vi "RunTest.vi"(8 "error in (no error)":errorcluster, 11 "Prueba04 in":refnum<class "Prueba04.lvclass">) -> (0 "error out":errorcluster, 2 "resultado":string, 3 "Prueba04 out":refnum<class "Prueba04.lvclass">)   [LabVIEW 2019, in "Prueba04.lvclass"]
uses:
  Prueba04.lvclass
  Control/Slide.ctl
  Prueba04.lvclass/Prueba04.ctl
  Control/SetPointGEN.ctl
  <vilib>/Utility/error.llb/DialogType.ctl
  QMH/Message Queue/Enqueue Message (Single).vi
  <vilib>/Utility/error.llb/Error Cluster From Error Code.vi
  <vilib>/ErrorRing/Error Ring.xnode
  Prueba/Prueba.lvclass
  QMH/User Event - Stop/User Event - Stop.lvlib
  QMH/Message Queue/Message Queue.lvlib
panel:
  out "frecZ1":dbl
  out "frecC1":dbl
  out "fila actual Z":i32
  out "frec_generar_Z2":string
  out "volt_generar_Z2":string
  out "frec_ref_Z_2":string="inicio"
  out "Vref_Z":dbl
  out "IndicadorAjuste_Z":dbl caption="Ajuste de amplitud [mV]"
  out "cumple_no_cumple_Z":bool
  out "cumple_no_cumple_C":bool
  out "fila actual C":i32
  out "frec_generar_C2":string
  out "volt_generar_C2":string
  out "frec_ref_C":string="inicio"
  out "IndicadorAjuste_C":dbl caption="Ajuste de amplitud [mV]"
  out "Vref_C":dbl
  out "cumple_no_cumple_A":bool
  out "ponderacion_Z":bool
  out "ponderacion_C":bool
  out "volt_generar_A2":string
  out "Vref_A 2":dbl
  out "frecA1":dbl
  out "frec_generar_C2":string
  out "Voltajes_Ref_Z":string[](array[string])
  out "Voltajes_Ref_C":string[](array[string])
  out "fila actual Z":i32
  out "fila actual C":i32
  out "frec_ref_Z":string="inicio"
  out "frec_ref_C":string="inicio"
  out "frec_generar_A2":string
  out "fila actual A":i32
  out "Voltajes_Ref_A":string[](array[string])
  out "frec_ref_A":string="inicio"
  out "Vref_A":dbl
  out "IndicadorAjuste_A":dbl caption="Ajuste de amplitud [mV]"
  out "ponderacion_A":bool
  out "Tab":T1(tab)
  in  "go_A":bool
  in  "go_C":bool
  in  "go_Z":bool
  in  "seguir":bool
  out "no_cumple_prueba04":bool
  out "cumple_prueba04":bool
  out "estado_ensayo_A":string="Ensayo ya realizado"
  out "estado_ensayo_C":string="Ensayo ya realizado"
  out "estado_ensayo_Z":string="Ensayo ya realizado"
  in  "cb_frec_A_1":string(combo)="1000"
  in  "guardar_Vref_A":bool
  out "niveldBA_1":dbl=95.0
  out "rangoRefA_1":dbl=140.0
  in  "generarA1":bool
  in  "VoltAjuste_A":T2=20.0 caption="Ajuste de amplitud [mV]" scale=0.0..50.0
  out "voltMonA_1":dbl format="%.5f"
  out "frecMonA_1":dbl format="%#.1f"
  in  "ir a resultados_A":bool
  out "Pict Ring_2":u16(ring)
  out "Pict Ring_1":u16(ring)
  in  "cb_frec_A_2":string(combo)="31,5"
  out "voltaje_A":dbl
  in  "generarA2":bool
  out "cumple_A":bool
  out "no_cumple_A":bool
  in  "ir a inicio desde A":bool
  in  "Tabla_A":string[][](table)
  out "voltMonA_2":dbl format="%.5f"
  out "frecMonA_2":dbl format="%#.1f"
  in  "cb_frec_C_1":string(combo)="1000"
  in  "guardar_Vref_C":bool
  out "niveldBC_1":dbl
  out "rangoRefC_1":dbl
  in  "generarC1":bool
  in  "VoltAjuste_C":T2=20.0 caption="Ajuste de amplitud [mV]" scale=0.0..50.0
  out "voltMonC_1":dbl
  out "frecMonC_1":dbl
  in  "ir a resultados_C":bool
  in  "cb_frec_C_2":string(combo)="31,5"
  out "voltaje_C":dbl
  in  "generarC2":bool
  out "voltMonC_2":dbl
  out "frecMonC_2":dbl
  in  "Tabla_C":string[][](table)
  in  "ir a inicio desde C":bool
  out "cumple_C":bool
  out "no_cumple_C":bool
  out "Pict Ring_1 2":u16(ring)
  out "Pict Ring_2 2":u16(ring)
  in  "cb_frec_Z_1":string(combo)="1000"
  out "niveldBZ_1":dbl
  out "rangoRefZ_1":dbl
  in  "generarZ1":bool
  in  "VoltAjuste_Z":T2=20.0 caption="Ajuste de amplitud [mV]" scale=0.0..200.0
  out "voltMonZ_1":dbl
  out "frecMonZ_1":dbl
  in  "ir a resultados _Z":bool
  in  "guardar_Vref_Z":bool
  out "Pict Ring_2 3":u16(ring)
  out "Pict Ring_1 3":u16(ring)
  in  "cb_frec_Z_2":string(combo)="31,5"
  out "voltaje_Z":dbl
  in  "generarZ2":bool
  in  "ir a inicio desde Z":bool
  in  "Tabla_Z":string[][](table)
  out "voltMonZ_2":dbl
  out "frecMonZ_2":dbl
  out "cumple_Z":bool
  out "no_cumple_Z":bool
  # "Cumple"
  # "No Cumple"
  # "Ensayo Eléctrico Ponderación A"
  # "Ensayo Eléctrico Ponderación C"
  # "Ensayo Eléctrico Ponderación Z"
  # "Ensayo Eléctrico Ponderación A – Selección de Señal de referencia"
  # "Elección Señal de Referencia\nsegún marca y modelo de sonómetro"
  # "Nivel en dB"
  # "Rango Referencia"
  # "Frecuencia"
  # "Monitoreo"
  # "Frecuencia"
  # "Hz"
  # "Voltaje"
  # "V"
  # "Ensayo Eléctrico Ponderación A – Tabla de Resultados"
  # "Cumple"
  # "No Cumple"
  # "Hz"
  # "mV"
  # "Voltaje"
  # "Frecuencia"
  # "Ponderación A"
  # "Monitoreo"
  # "Frecuencia"
  # "Hz"
  # "Voltaje"
  # "V"
  # "Ensayo Eléctrico Ponderación C – Selección de Señal de referencia"
  # "Elección Señal de Referencia\nsegún marca y modelo de sonómetro"
  # "Nivel en dB"
  # "Rango Referencia"
  # "Frecuencia"
  # "Monitoreo"
  # "Frecuencia"
  # "Hz"
  # "Voltaje"
  # "V"
  # "Ensayo Eléctrico Ponderación C – Tabla de Resultados"
  # "Cumple"
  # "No Cumple"
  # "Hz"
  # "mV"
  # "Voltaje"
  # "Frecuencia"
  # "Monitoreo"
  # "Frecuencia"
  # "Hz"
  # "Voltaje"
  # "V"
  # "Ponderación C"
  # "Ensayo Eléctrico Ponderación Z – Selección de Señal de referencia"
  # "Elección Señal de Referencia\nsegún marca y modelo de sonómetro"
  # "Nivel en dB"
  # "Rango Referencia"
  # "Frecuencia"
  # "Monitoreo"
  # "Frecuencia"
  # "Hz"
  # "Voltaje"
  # "V"
  # "Ensayo Eléctrico Ponderación Z – Tabla de Resultados"
  # "Cumple"
  # "No Cumple"
  # "Hz"
  # "mV"
  # "Voltaje"
  # "Frecuencia"
  # "Ponderación Z"
  # "Monitoreo"
  # "Frecuencia"
  # "Hz"
  # "Voltaje"
  # "V"
  # "4. Ensayo  de las ponderaciones frecuenciales con señales eléctricas. IEC 61672-3: 2006 Cláusula 12"
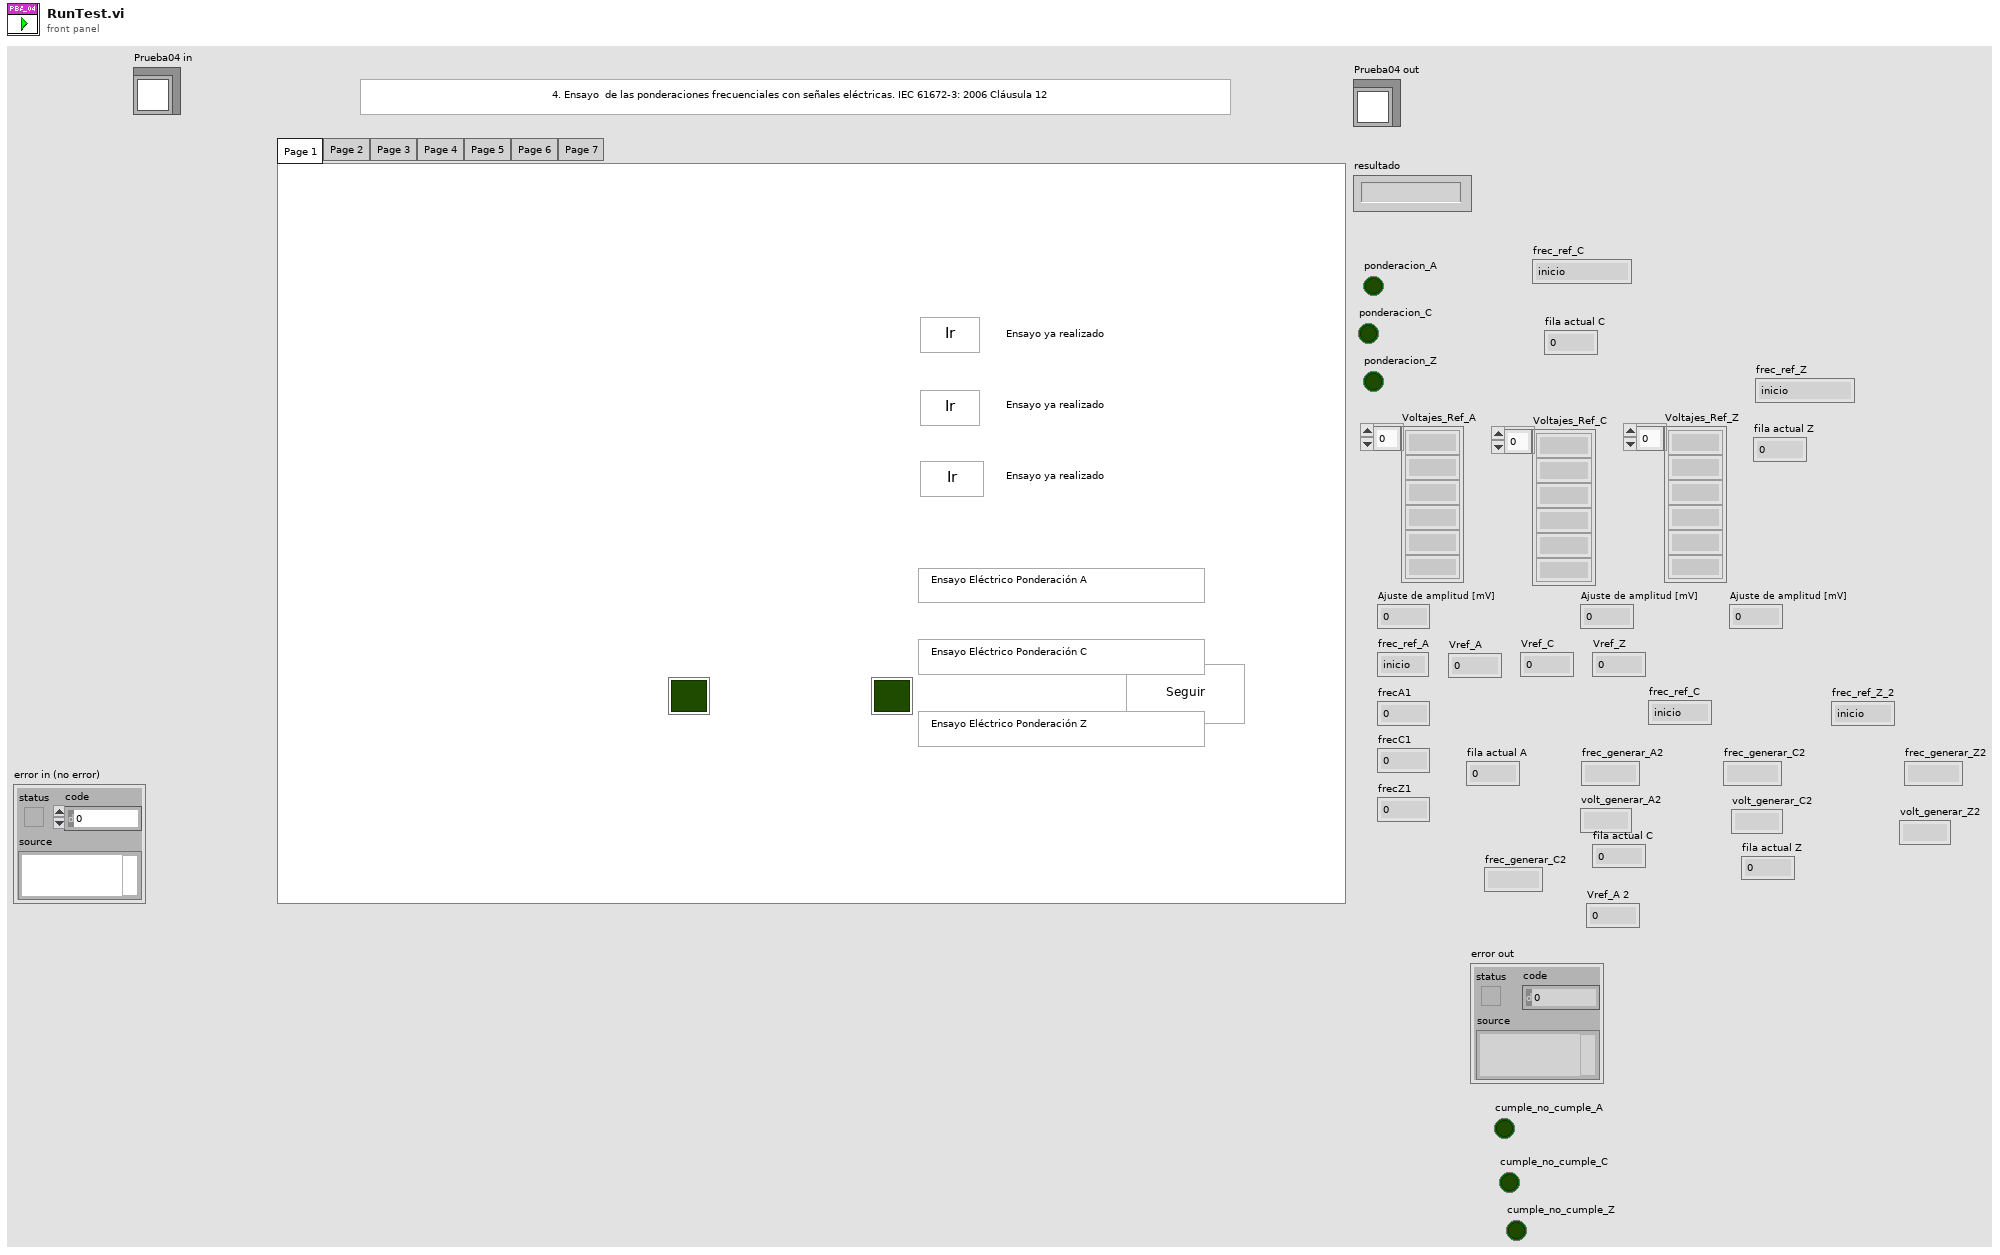
[diagram p1: front panel]
types:
  T1 = enum32{"Page 1", "Page 2", "Page 3", "Page 4", "Page 5", "Page 6", "Page 7"}
  T2 = typedef "Prueba04.lvclass/Slide.ctl" = dbl
  T3 = enum8{"Enabled", "Disabled", "Disabled and Grayed Out"}
  T4 = typedef "Message Queue.lvlib/All Message Queues.ctl" = cluster{"MHL":refnum<queue>, "Inst_CNT90":refnum<queue>, "Inst_DS360":refnum<queue>, "Inst_Keithley2002":refnum<queue>, "Inst_DAQ":refnum<queue>, "BD":refnum<queue>, "Pistofono":refnum<queue>, "Nexus":refnum<queue>}
  T5 = typedef "Prueba04.lvclass/SetPointGEN.ctl" = cluster{"frec":dbl, "amp":dbl, "letra":string}
  T6 = cluster{"ControlName":string, "ControlReference":refnum<vi>}[]
  T7 = cluster{"Medido":dbl, "Error":dbl, "Ref":dbl, "Incert_exp":dbl, "Tol+":dbl, "Tol-":dbl, "fila":i32}
  T8 = typedef "DialogType.ctl" = u16
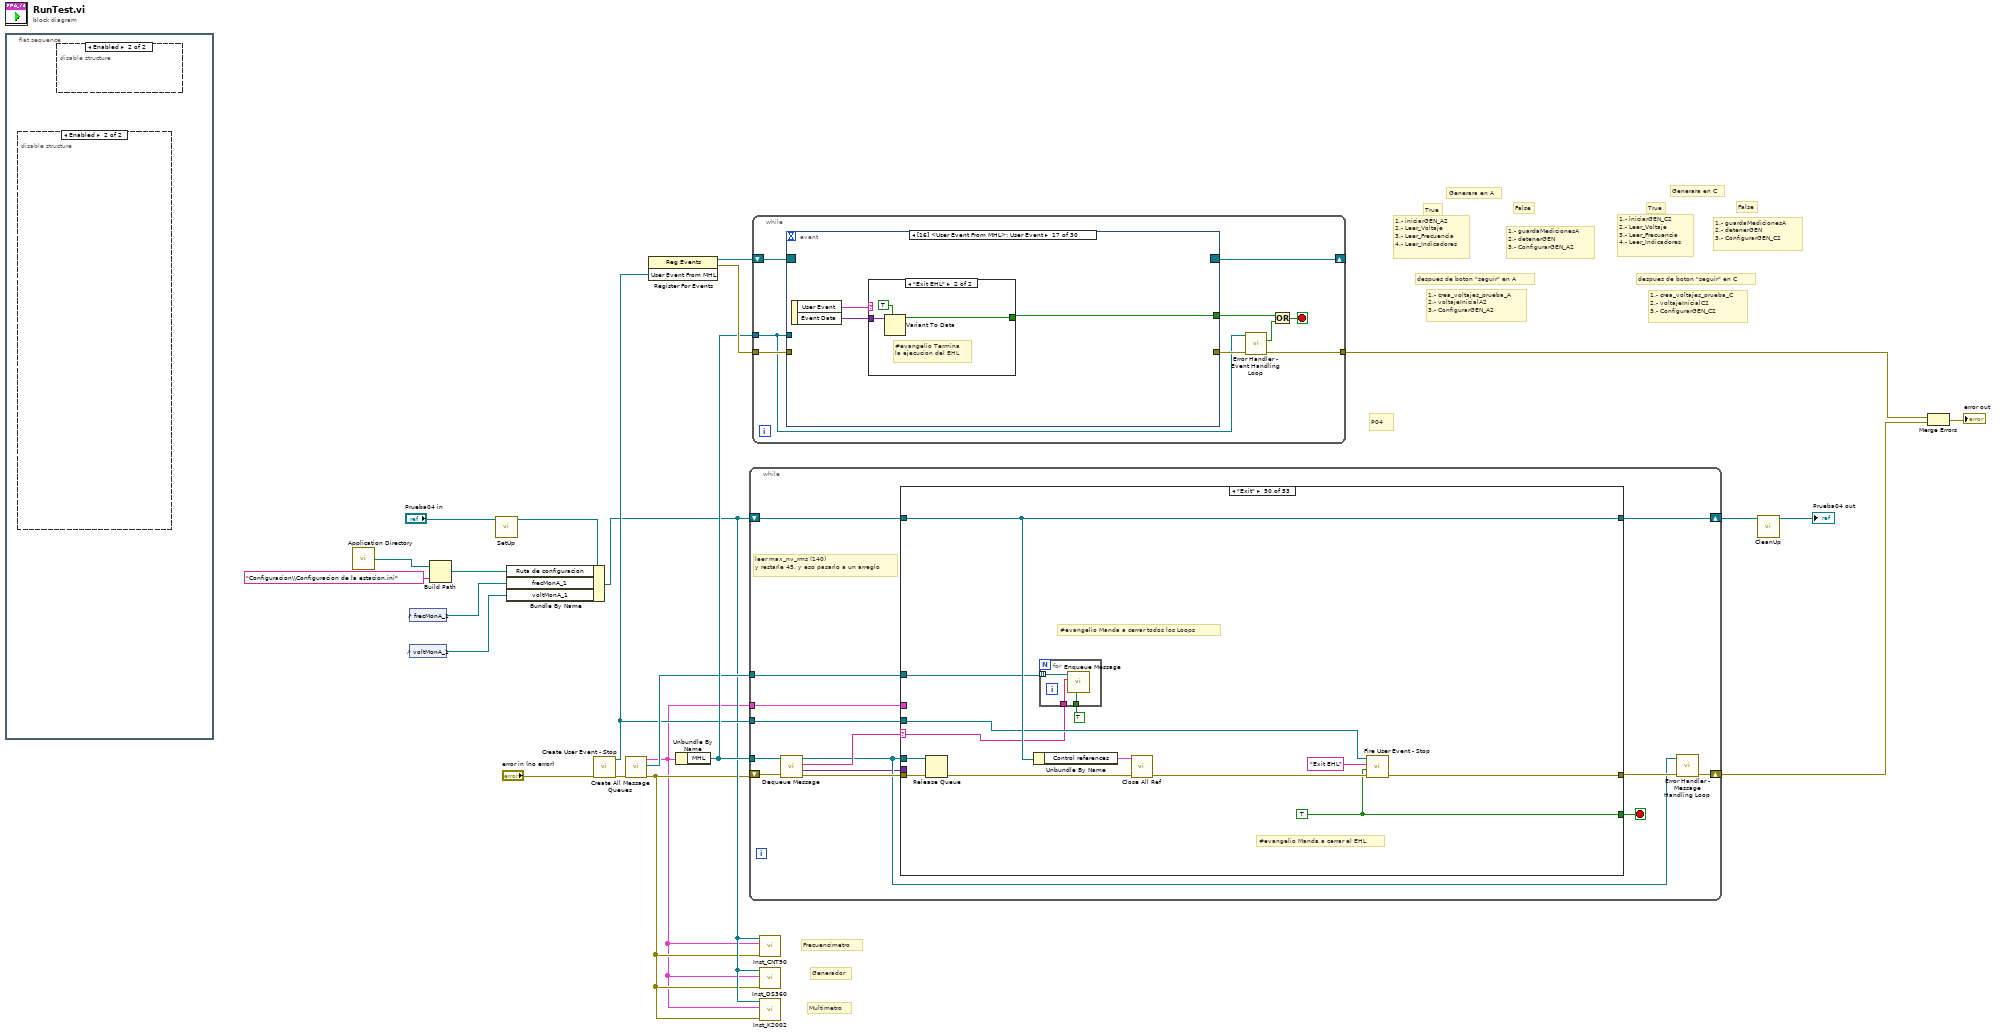
[diagram p0: block diagram]
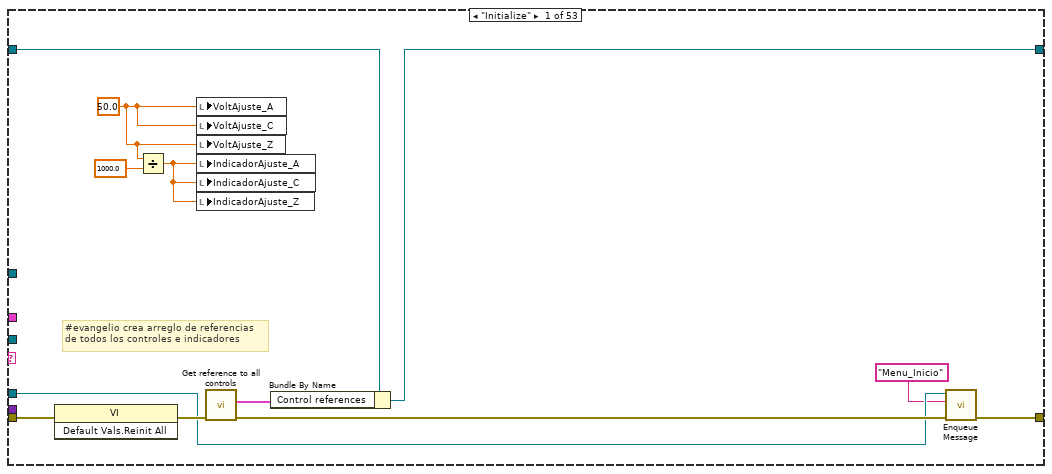
[diagram p2: hidden frame]
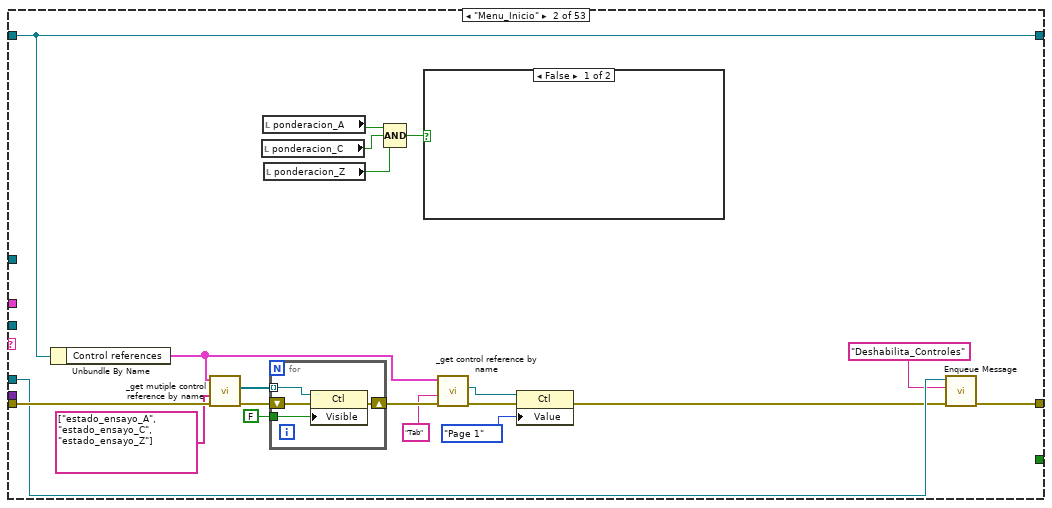
[diagram p3: hidden frame]
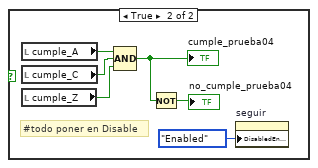
[diagram p4: hidden frame]
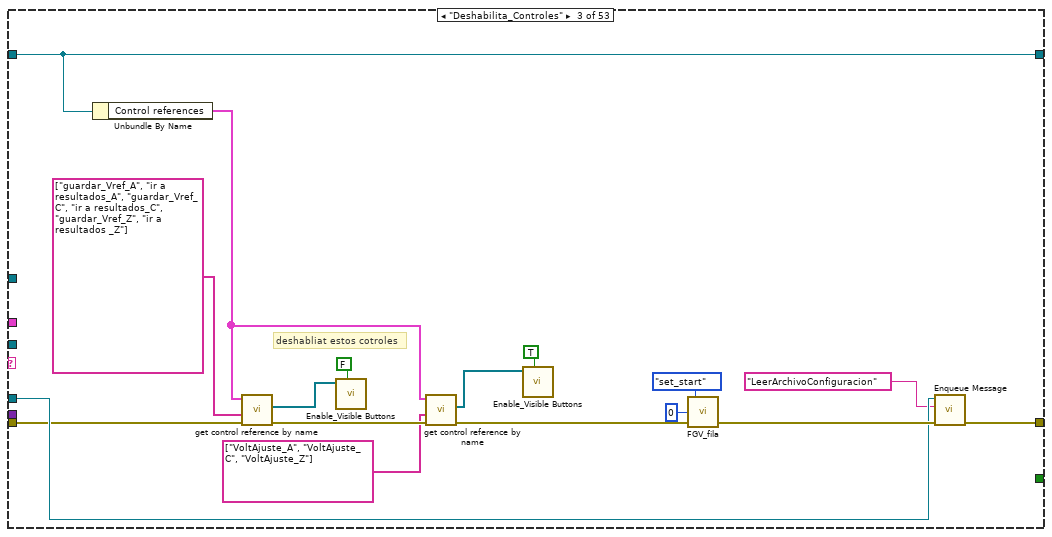
[diagram p5: hidden frame]
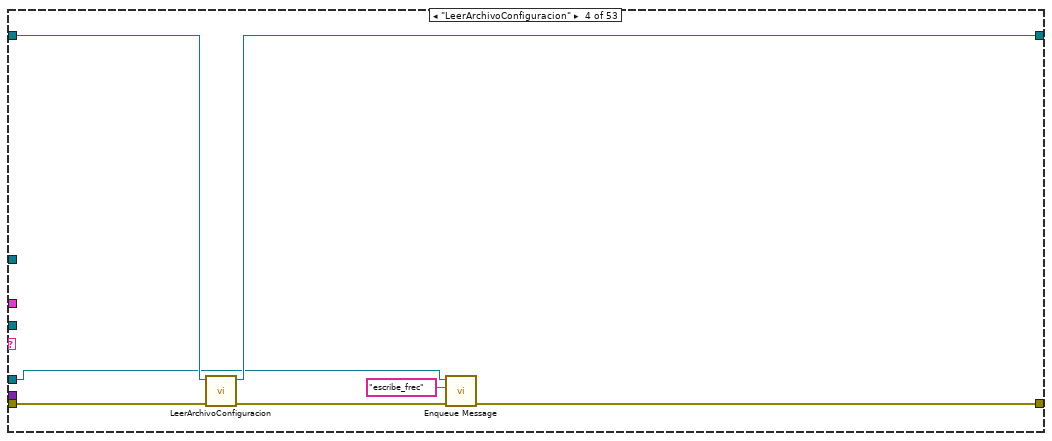
[diagram p6: hidden frame]
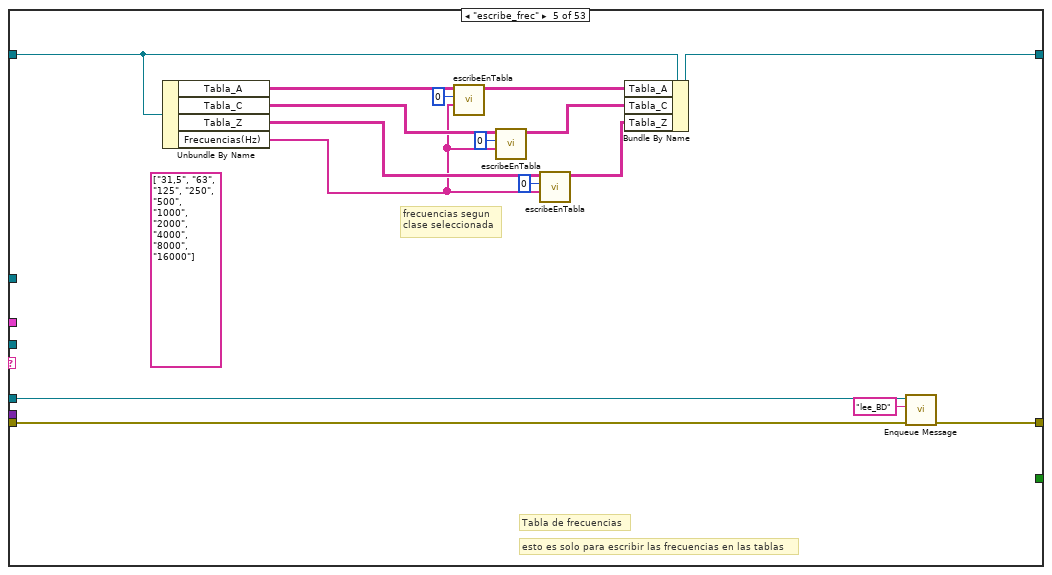
[diagram p7: hidden frame]
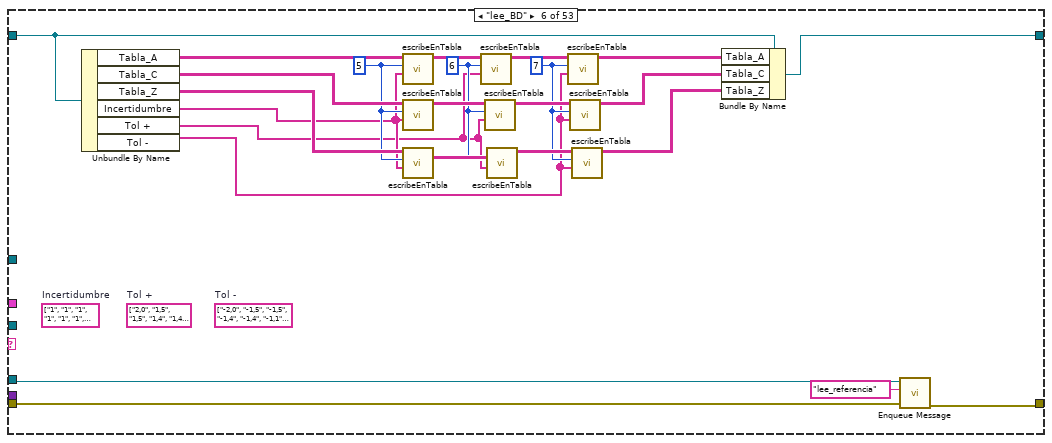
[diagram p8: hidden frame]
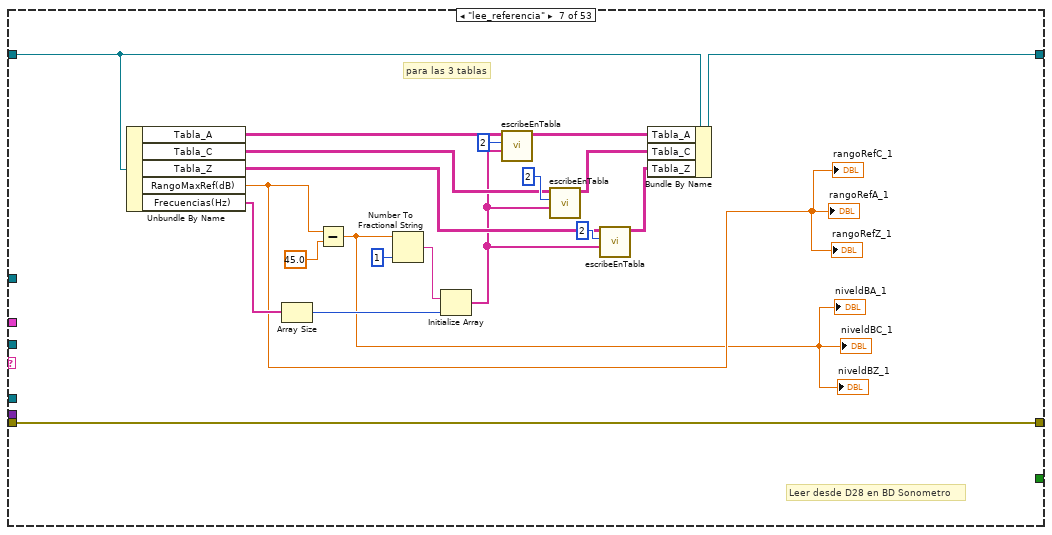
[diagram p9: hidden frame]
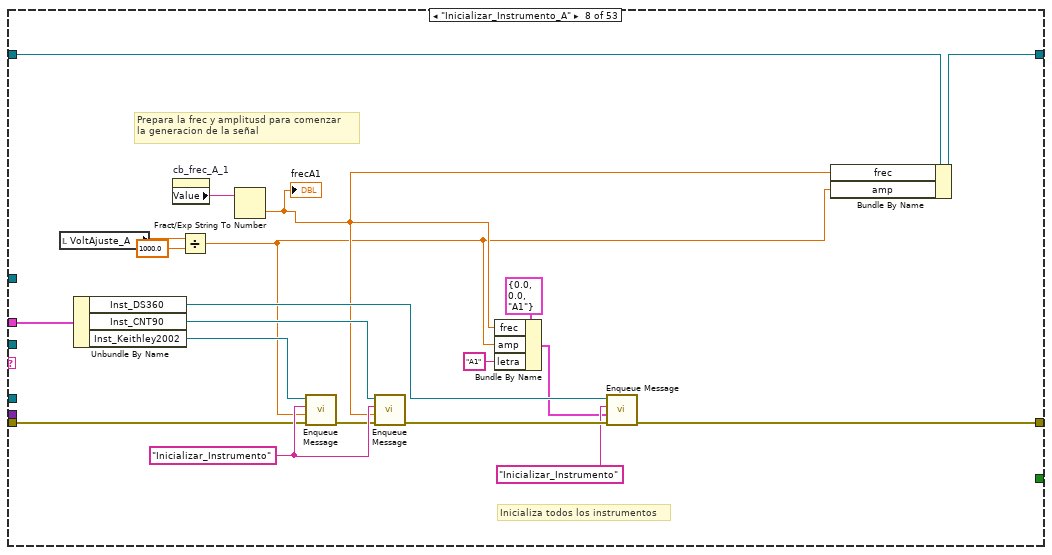
[diagram p10: hidden frame]
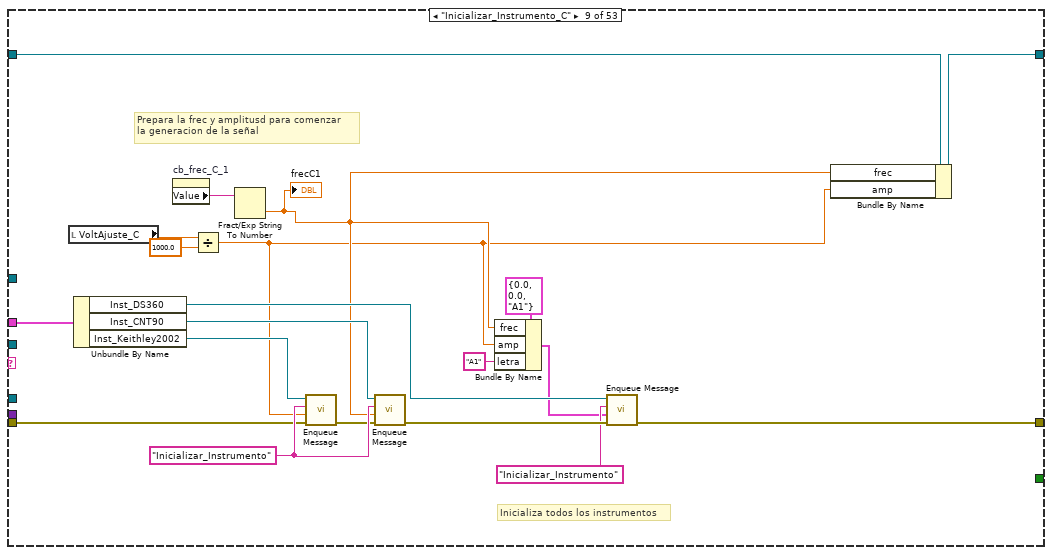
[diagram p11: hidden frame]
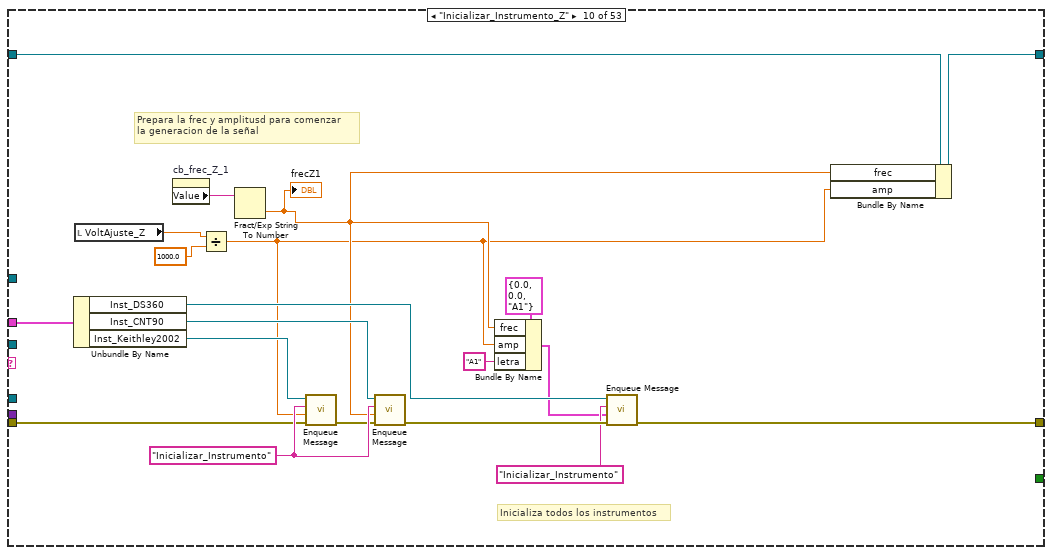
[diagram p12: hidden frame]
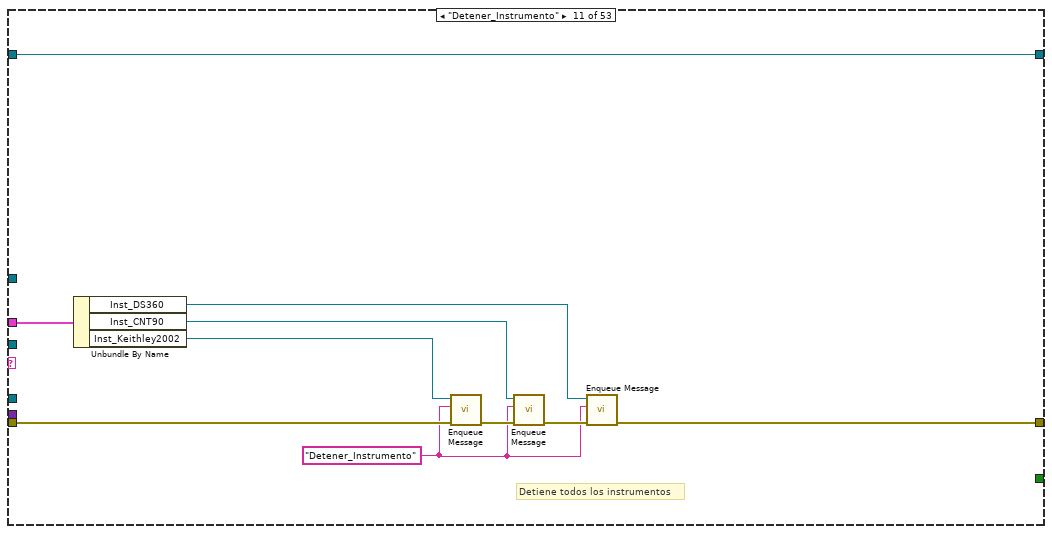
[diagram p13: hidden frame]
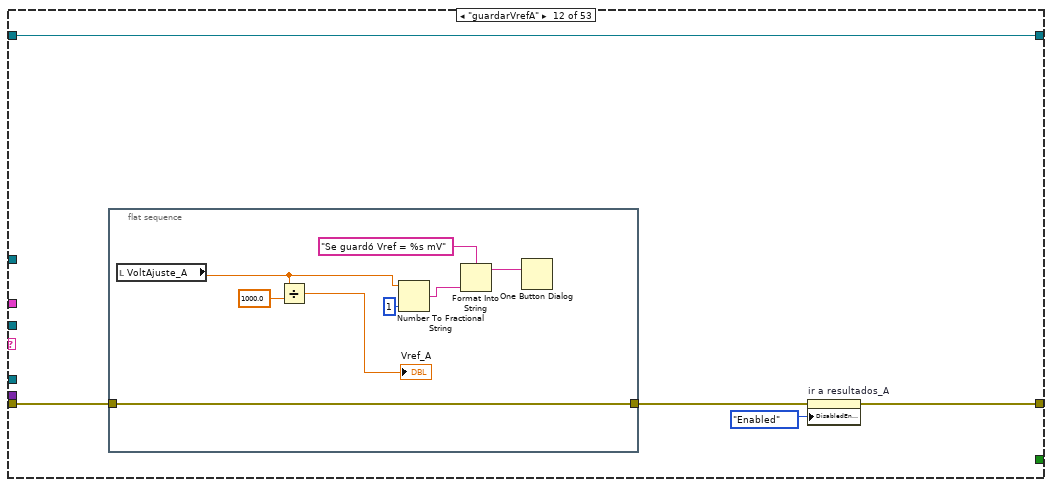
[diagram p14: hidden frame]
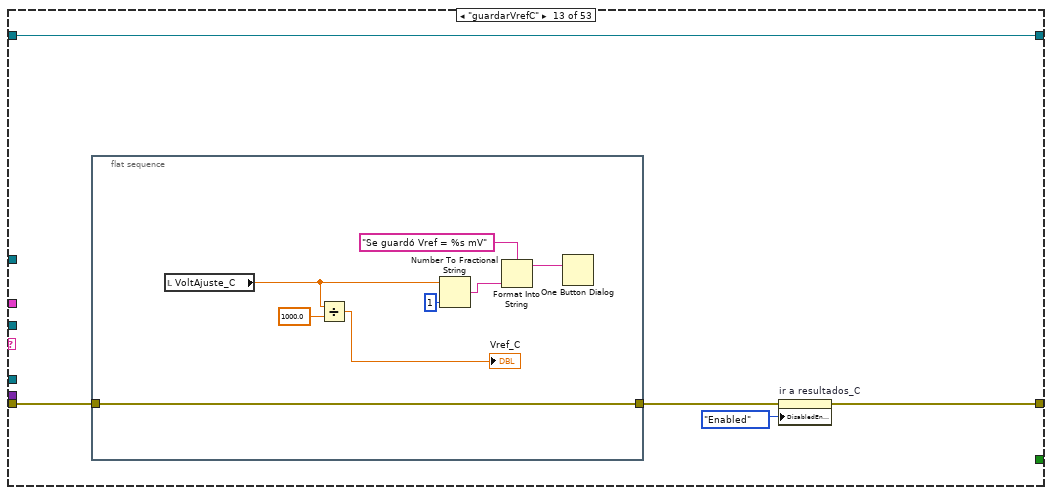
[diagram p15: hidden frame]
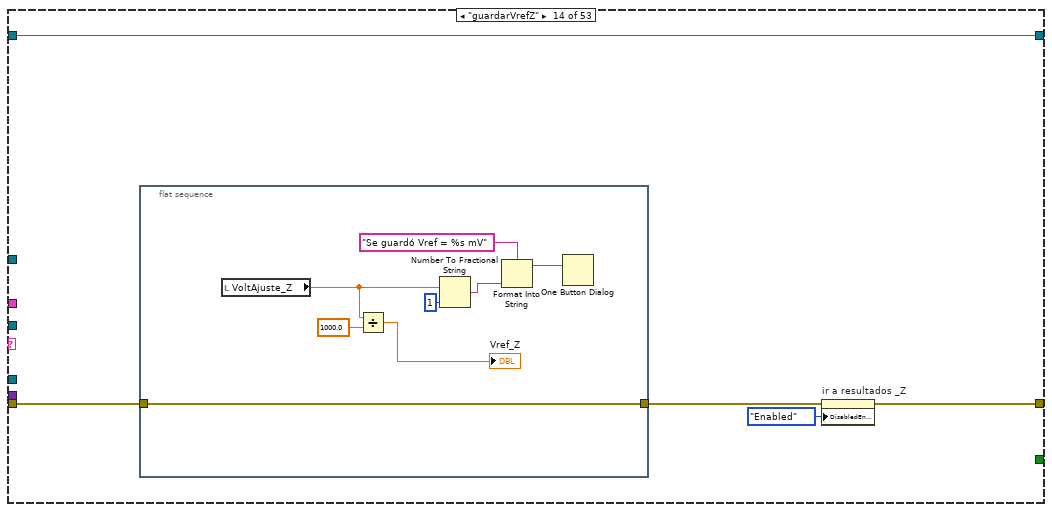
[diagram p16: hidden frame]
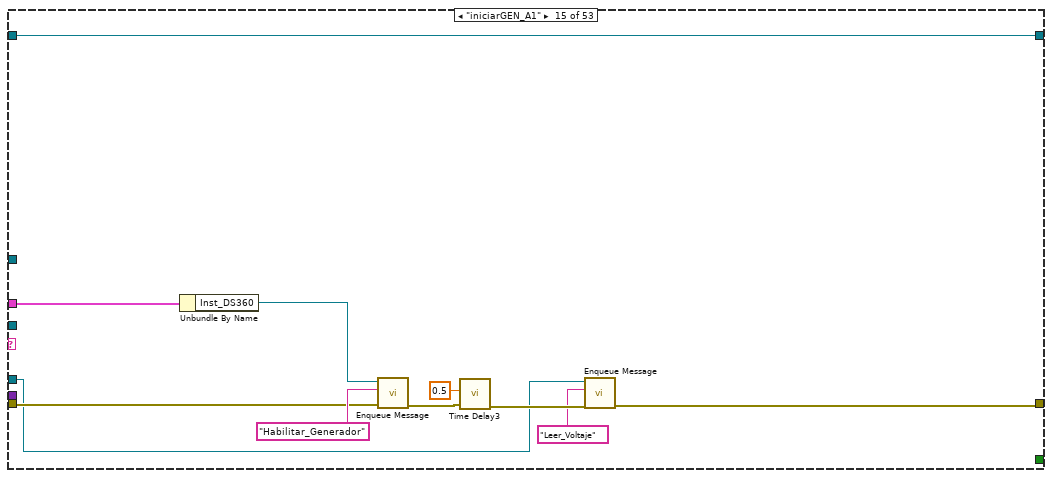
[diagram p17: hidden frame]
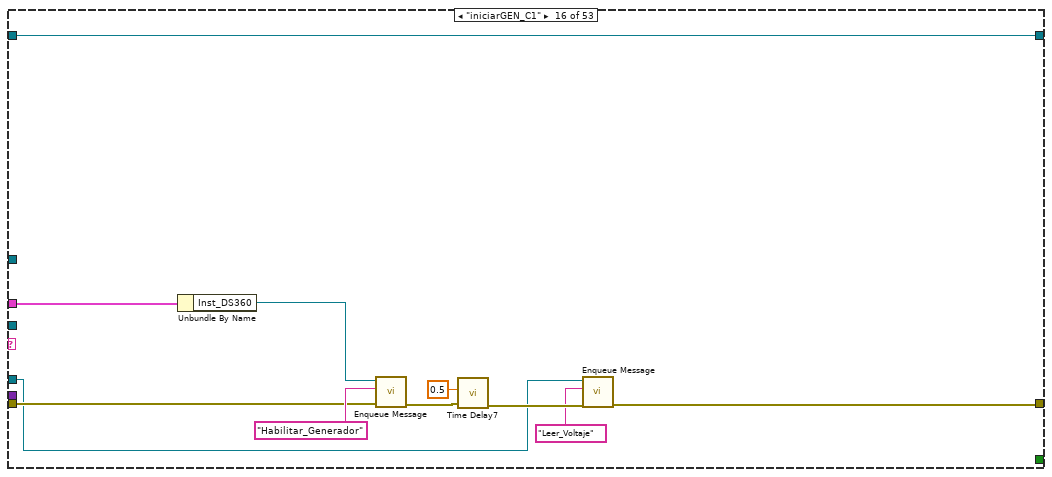
[diagram p18: hidden frame]
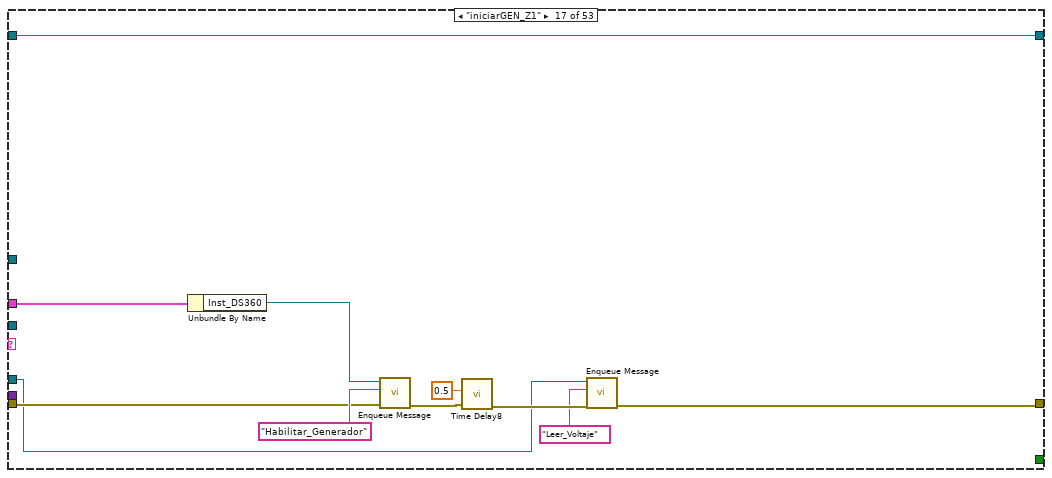
[diagram p19: hidden frame]
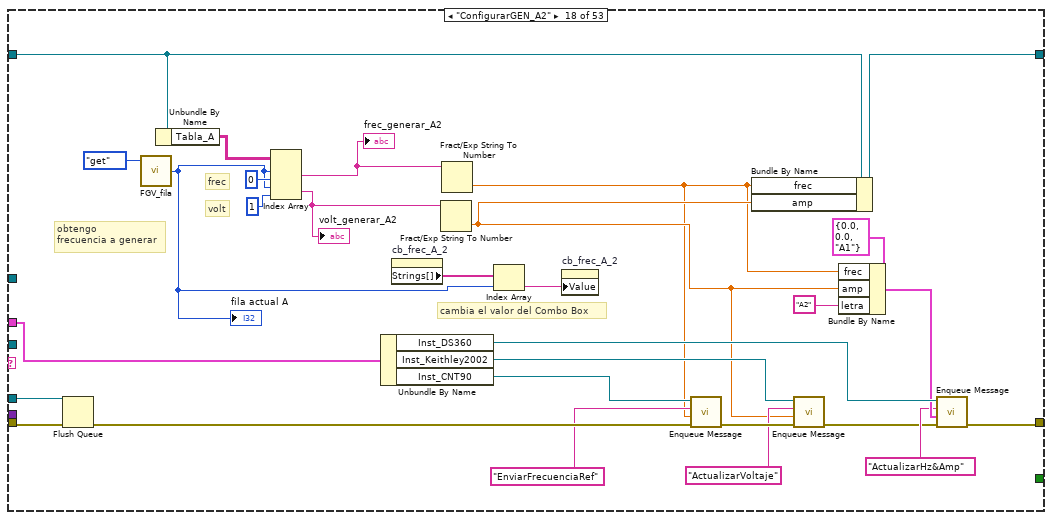
[diagram p20: hidden frame]
diagram:
  # "despues de boton \"seguir\" en C"
  # "1.- crea_voltajes_prueba_C\n2.- voltajeInicialC2\n3.- ConfigurarGEN_C2"
  # "1.- guardaMedicionesA\n2.- detenerGEN\n3.- ConfigurarGEN_A2"
  # "False"
  # "True"
  # "1.- iniciarGEN_A2\n2.- Leer_Voltaje\n3.- Leer_Frecuencia\n4.- Leer_Indicadores"
  # "Generara en A"
  # "1.- guardaMedicionesA\n2.- detenerGEN\n3.- ConfigurarGEN_C2"
  # "False"
  # "True"
  # "1.- iniciarGEN_C2\n2.- Leer_Voltaje\n3.- Leer_Frecuencia\n4.- Leer_Indicadores"
  # "Generara en C"
  # "despues de boton \"seguir\" en A"
  # "1.- crea_voltajes_prueba_A\n2.- voltajeInicialA2\n3.- ConfigurarGEN_A2"
  # "P04"
  # "Multimetro"
  # "Generador"
  # "Frecuencimetro"
  n1 = flat-sequence {
    frame #0 {
      n2 = disable-structure shown="Enabled" {
        frame Disabled {
          w24 = FALSE ("cumple_A")
          n3 = local write "generarA1"(w24) -> ()
          n4 = local write "no_cumple_A"(w24) -> ()
          n5 = local write "cumple_prueba04"(w24) -> ()
          n6 = local write "no_cumple_prueba04"(w24) -> ()
          n7 = local write "generarA2"(w24) -> ()
          n8 = local write "generarZ1"(w24) -> ()
          n9 = local write "no_cumple_Z"(w24) -> ()
          n10 = local write "generarC1"(w24) -> ()
          n11 = local write "no_cumple_C"(w24) -> ()
          n12 = local write "generarC2"(w24) -> ()
          n13 = local write "generarZ2"(w24) -> ()
          n14 = local write "ponderacion_A"(w24) -> ()
          n15 = local write "ponderacion_C"(w24) -> ()
          n16 = local write "ir a inicio desde C"(w24) -> ()
          n17 = local write "ponderacion_Z"(w24) -> ()
          n18 = local write "cumple_A"(w24) -> ()
          n19 = local write "cumple_C"(w24) -> ()
          n20 = local write "cumple_Z"(w24) -> ()
          n21 = local write "ir a inicio desde A"(w24) -> ()
          n22 = local write "ir a inicio desde Z"(w24) -> ()
        }
        frame Enabled {
        }
      }
      n23 = disable-structure shown="Enabled" {
        frame Disabled {
          n24 = property on="seguir" class="Bool"("DisabledEnum"=T3."Enabled" ("Disabled")) -> ()  [unwired: 2 in, 2 out]
        }
        frame Enabled {
        }
      }
    }
  }
  n25 = call <vilib>:"Application Directory.vi"() -> ("Application Directory"=w16:path)
  n26 = control-ref of="frecMonA_1"() -> (w2:refnum<vi>)
  n27 = control-ref of="voltMonA_1"() -> (w1:refnum<vi>)
  n28 = Build Path(base path=w16, name or relative path="Configuracion\\Configuracion de la estacion.ini") -> (appended path=w15:path)
  n29 = call-dynamic "SetUp.vi"("Prueba04 in"="Prueba04 in") -> ("Prueba04 out"=w14:refnum<class "Prueba04.lvclass">)  [unwired: 9 in, 1 out]
  n30 = Bundle By Name(cluster=w14, "Ruta de configuracion"=w15, "frecMonA_1"=w2, "voltMonA_1"=w1) -> (w5:refnum<class "Prueba04.lvclass">)
  n31 = call "Create User Event - Stop.vi"("error in (no error)"="error in (no error)") -> ("error out"=w13:errorcluster, "User Event From MHL"=w6:refnum<user-event>)  [unwired: 9 in]
  n32 = call "Create All Message Queues.vi"("error in (no error)"=w13) -> ("error out"=w4:errorcluster, "PL Queues Array"=w7:refnum<queue>[], "All Message Queues out"=w3:T4)  [unwired: 8 in]
  n33 = register-events(w6) -> (reference out=w18:refnum<event-registration>, error out=w11:errorcluster)  [unwired: 2 in]
  n34 = Unbundle By Name(w3) -> ("MHL"=w10:refnum<queue>)
  n35 = while {
    shift-right: [w35] -> w19
    shift-left: w5 -> [w36]
    shift-right: [w30] -> w21
    shift-left: w4 -> [w34]
    tunnel: w10 -> [w33]
    tunnel: w7 -> [w27]
    tunnel: w3 -> [w26]
    tunnel: w6 -> [w25]
    stop <- w37 stop-if-true
    # "leer max_nv_rms (140)\ny restarle 45, y eso pasarlo a un arreglo"
    n36 = call "Dequeue Message.vi"("error in (no error)"=w34, "Message Queue"=w33) -> ("error out"=w38:errorcluster, "Message Data"=w28:variant, "Message"=w32:string, "dup Message Queue"=w29:refnum<queue>)  [unwired: 6 in]
    n37 = case shown="\"Exit\"" w32 {
      selector: w32 -> [_ _ _ _ _ _ _ _ _ _ _ _ _ _ _ _ _ _ _ _ _ _ _ _ _ _ _ _ _ _ _ _ _ _ _ _ _ _ _ _ _ _ _ _ _ _ _ _ _ w1001 _ w1026 _]
      tunnel: [_ _ _ _ _ _ _ _ _ _ _ _ _ _ _ _ _ _ _ _ _ _ _ _ _ _ _ _ _ _ _ _ _ _ _ _ _ _ _ _ _ _ _ _ _ _ _ _ _ w1000 _ _ _] -> w37
      tunnel: [w47 w69 w95 w100 w120 w144 w164 w173 w193 w213 w232 w235 w248 w261 w275 w286 w297 w322 w348 w375 w393 w405 w417 w428 w441 w459 w468 w494 w500 w522 w545 w568 w578 w590 w602 w611 w620 w627 w646 w665 w684 w727 w814 w850 w863 w903 w943 w981 w983 w999 w1016 w1025 w1036] -> w31
      tunnel: w38 -> [w49 w70 w91 w104 w119 w143 w164 w170 w190 w210 w234 w238 w251 w264 w277 w288 w299 w329 w356 w385 w396 w408 w420 w431 w444 w461 w470 w486 w507 w531 w554 w570 w581 w591 w603 w612 w621 w637 w656 w675 w695 w728 w815 w850 w864 w904 w944 w978 w984 w1006 w1018 _ w1036]
      tunnel: w36 -> [w46 w56 w90 w103 w108 w142 w161 w183 w203 w223 w233 w239 w252 w265 w284 w295 w306 w327 w353 w383 w403 w415 w427 w440 w453 w458 w483 w493 w503 w525 w548 w569 w579 w589 w597 w606 w615 w635 w654 w673 w689 w723 w810 w843 w859 w899 w939 w976 w990 w1004 w1024 w1027 w1035]
      tunnel: [w45 w56 w90 w102 w112 w138 w162 w182 w202 w222 w233 w239 w252 w265 w284 w295 w306 w328 w354 w384 w403 w415 w427 w440 w453 w458 w483 w493 w505 w527 w550 w569 w579 w589 w597 w606 w615 w633 w652 w671 w690 w723 w810 w843 w857 w897 w937 w976 w990 w1004 w1024 w1027 w1035] -> w35
      tunnel: w29 -> [w44 w68 w93 w99 w106 w122 _ _ _ _ _ _ _ _ w274 w285 w296 w323 w349 w379 w394 w406 w418 w430 w443 w460 _ _ w501 w523 w546 w567 w577 w587 _ _ _ w629 w648 w667 w683 w721 w808 _ w853 w893 w933 w975 w985 w1005 w1017 _ _]
      tunnel: w28 -> [_ _ _ _ _ _ _ _ _ _ _ _ _ _ _ _ _ _ _ _ _ _ _ _ _ _ w467 _ _ _ _ _ _ _ _ _ _ w628 w647 w666 w685 w722 w809 _ _ _ _ _ _ _ w1015 _ _]
      tunnel: w27 -> [_ _ _ _ _ _ _ _ _ _ _ _ _ _ _ _ _ _ _ _ _ _ _ _ _ _ _ _ _ _ _ _ _ _ _ _ _ _ _ _ _ _ _ _ _ _ _ _ _ w1003 _ _ _]
      tunnel: w26 -> [_ _ _ _ _ _ _ w181 w201 w221 w231 _ _ _ w276 w287 w298 w321 w347 w374 w395 w407 w419 w429 w442 _ w469 w485 _ _ _ _ _ _ _ _ _ _ _ _ _ _ _ _ _ _ _ _ _ _ _ _ _]
      tunnel: w25 -> [_ _ _ _ _ _ _ _ _ _ _ _ _ _ _ _ _ _ _ _ _ _ _ _ _ _ _ _ _ _ _ _ _ _ _ _ _ _ _ _ _ _ _ _ _ _ _ _ _ w1002 _ _ _]
      frame "Initialize" {
        w39 = T2 50.0 ("VoltAjuste_A")
        # "#evangelio crea arreglo de referencias\nde todos los controles e indicadores"
        n38 = invoke class="VI" method="Default Vals.Reinit All"(error in=w49) -> (error out=w50:errorcluster)  [unwired: 2 in, 2 out]
        n39 = Divide(x=w39, y=T2 1000.0) -> (x/y=w41:T2)
        n40 = local write "VoltAjuste_A"(w39) -> ()
        n41 = local write "VoltAjuste_C"(w39) -> ()
        n42 = local write "VoltAjuste_Z"(w39) -> ()
        n43 = local write "IndicadorAjuste_A"(w41) -> ()
        n44 = local write "IndicadorAjuste_C"(w41) -> ()
        n45 = local write "IndicadorAjuste_Z"(w41) -> ()
        n46 = call "Get reference to all controls.vi"("error in (no error)"=w50) -> ("error out"=w48:errorcluster, "Control references"=w42:T6)  [unwired: 5 in]
        n47 = Bundle By Name(cluster=w46, "Control references"=w42) -> (w45:refnum<class "Prueba04.lvclass">)
        n48 = call-poly "Enqueue Message.vi"("error in (no error)"=w48, "Message"="Menu_Inicio", "Message Queue"=w44) -> ("error out"=w47:errorcluster)  [unwired: 7 in, 1 out]
      }
      frame "Menu_Inicio" {
        n49 = Unbundle By Name(w56) -> ("Control references"=w55:T6)
        n50 = call "_get mutiple control reference by name.vi"("error in (no error)"=w70, "Control names"=string[] ["estado_ensayo_A", "estado_ensayo_C", "estado_ensayo_Z"], "Control references"=w55) -> ("error out"=w66:errorcluster, "References"=w64:refnum<vi>[])  [unwired: 3 in]
        n51 = local read "ponderacion_C"() -> (w52:bool)
        n52 = local read "ponderacion_A"() -> (w53:bool)
        n53 = local read "ponderacion_Z"() -> (w54:bool)
        n54 = for {
          shift-right: [w79] -> w62
          shift-left: w66 -> [w80]
          tunnel: w64 -> [w78] mode=indexing
          tunnel: FALSE -> [w77]
          n55 = property class="Ctl"(reference=w78, error in=w80, "Visible"=w77) -> (error out=w79:errorcluster)  [unwired: 1 out]
        }
        n56 = Compound Arithmetic op=AND(w53, w52, w54) -> (w51:bool)
        n57 = case shown="False" w51 {
          frame False {
          }
          frame True {
            # "#todo poner en Disable"
            n58 = local read "cumple_A"() -> (w76:bool)
            n59 = local read "cumple_C"() -> (w72:bool)
            n60 = local read "cumple_Z"() -> (w71:bool)
            n61 = Compound Arithmetic op=AND(w76, w72, w71) -> (w73:bool)
            "cumple_prueba04" <- w73
            n62 = Not(x=w73) -> (.not. x?=→"no_cumple_prueba04":bool)
            n63 = property on="seguir" class="Bool"("DisabledEnum"=T3."Enabled" ("Disabled")) -> ()  [unwired: 2 in, 2 out]
          }
        }
        n64 = call "_get control reference by name.vi"("error in (no error)"=w62, "Control name"="Tab" ("Message"), "Control references"=w55) -> ("error out"=w61:errorcluster, "Ctl Refnum"=w58:refnum<vi>)  [unwired: 3 in]
        n65 = property class="Ctl"(reference=w58, error in=w61, "Value"=T1."Page 1" ("Tab_Prueba04")) -> (error out=w59:errorcluster)  [unwired: 1 out]
        n66 = call-poly "Enqueue Message.vi"("error in (no error)"=w59, "Message"="Deshabilita_Controles", "Message Queue"=w68) -> ("error out"=w69:errorcluster)  [unwired: 7 in, 1 out]
      }
      frame "Deshabilita_Controles" {
        # "deshabliat estos cotroles"
        n67 = Unbundle By Name(w90) -> ("Control references"=w86:T6)
        n68 = call-poly "get control reference by name.vi"("error in (no error)"=w91, "Control names"=string[] ["guardar_Vref_A", "ir a resultados_A", "guardar_Vref_C", "ir a resultados_C", "guardar_Vref_Z", "ir a resultados _Z"] ("Message"), "Control references"=w86) -> ("error out"=w85:errorcluster, "References"=w88:refnum<vi>[])  [unwired: 3 in]
        n69 = call "Enable_Visible Buttons.vi"("Enable? (T)"=FALSE, "Controls Ref Array"=w88) -> ()  [unwired: 10 in]
        n70 = call-poly "get control reference by name.vi"("error in (no error)"=w85, "Control names"=string[] ["VoltAjuste_A", "VoltAjuste_C", "VoltAjuste_Z"] ("Message"), "Control references"=w86) -> ("error out"=w84:errorcluster, "References"=w81:refnum<vi>[])  [unwired: 3 in]
        n71 = call "Enable_Visible Buttons.vi"("Enable? (T)"=TRUE, "Controls Ref Array"=w81) -> ()  [unwired: 10 in]
        n72 = call "FGV_fila.vi"("error in (no error)"=w84, "fila_inicial"=0, "action"=enum16{"increment", "set_start", "get"}."set_start") -> ("error out"=w94:errorcluster)  [unwired: 1 in, 1 out]
        n73 = call-poly "Enqueue Message.vi"("error in (no error)"=w94, "Message"="LeerArchivoConfiguracion", "Message Queue"=w93) -> ("error out"=w95:errorcluster)  [unwired: 7 in, 1 out]
      }
      frame "LeerArchivoConfiguracion" {
        n74 = call "LeerArchivoConfiguracion.vi"("error in (no error)"=w104, "Prueba04 in"=w103) -> ("error out"=w101:errorcluster, "Prueba04 out"=w102:refnum<class "Prueba04.lvclass">)  [unwired: 8 in]
        n75 = call-poly "Enqueue Message.vi"("error in (no error)"=w101, "Message"="escribe_frec", "Message Queue"=w99) -> ("error out"=w100:errorcluster)  [unwired: 7 in, 1 out]
      }
      frame "escribe_frec" {
        (unwired) string[] ["31,5", "63", "125", "250", "500", "1000", "2000", "4000", "8000", "16000"]
        # "frecuencias segun\nclase seleccionada"
        # "esto es solo para escribir las frecuencias en las tablas"
        # "Tabla de frecuencias"
        n76 = Unbundle By Name(w108) -> ("Tabla_A"=w118:string[][], "Tabla_C"=w116:string[][], "Tabla_Z"=w115:string[][], "Frecuencias(Hz)"=w107:string[])
        n77 = call "escribeEnTabla.vi"("parametros"=w107, "col"=0, "tabla in"=w118) -> ("tabla out"=w111:string[][])  [unwired: 8 in]
        n78 = call "escribeEnTabla.vi"("parametros"=w107, "col"=0, "tabla in"=w116) -> ("tabla out"=w110:string[][])  [unwired: 8 in]
        n79 = call "escribeEnTabla.vi"("parametros"=w107, "col"=0, "tabla in"=w115) -> ("tabla out"=w109:string[][])  [unwired: 8 in]
        n80 = Bundle By Name(cluster=w108, "Tabla_A"=w111, "Tabla_C"=w110, "Tabla_Z"=w109) -> (w112:refnum<class "Prueba04.lvclass">)
        n81 = call-poly "Enqueue Message.vi"("error in (no error)"=w119, "Message"="lee_BD", "Message Queue"=w106) -> ("error out"=w120:errorcluster)  [unwired: 7 in, 1 out]
      }
      frame "lee_BD" {
        w126 = 7 ("col")
        w127 = 6 ("col")
        w128 = 5 ("col")
        (unwired) string[] ["-2,0", "-1,5", "-1,5", "-1,4", "-1,4", "-1,1", "-1,6", "-1,6", "-3,1", "-17,0"]  # Tol -
        (unwired) string[] ["2,0", "1,5", "1,5", "1,4", "1,4", "1,1", "1,6", "1,6", "2,1", "3,5"]  # Tol +
        (unwired) string[] ["1", "1", "1", "1", "1", "1", "1", "1", "1", "1"]  # Incertidumbre
        n82 = Unbundle By Name(w142) -> ("Tabla_A"=w141:string[][], "Tabla_C"=w140:string[][], "Tabla_Z"=w139:string[][], "Incertidumbre"=w125:string[], "Tol +"=w124:string[], "Tol -"=w123:string[])
        n83 = call "escribeEnTabla.vi"("parametros"=w125, "col"=w128, "tabla in"=w141) -> ("tabla out"=w137:string[][])  [unwired: 8 in]
        n84 = call "escribeEnTabla.vi"("parametros"=w125, "col"=w128, "tabla in"=w140) -> ("tabla out"=w133:string[][])  [unwired: 8 in]
        n85 = call "escribeEnTabla.vi"("parametros"=w125, "col"=w128, "tabla in"=w139) -> ("tabla out"=w130:string[][])  [unwired: 8 in]
        n86 = call "escribeEnTabla.vi"("parametros"=w124, "col"=w127, "tabla in"=w137) -> ("tabla out"=w134:string[][])  [unwired: 8 in]
        n87 = call "escribeEnTabla.vi"("parametros"=w124, "col"=w127, "tabla in"=w133) -> ("tabla out"=w132:string[][])  [unwired: 8 in]
        n88 = call "escribeEnTabla.vi"("parametros"=w124, "col"=w127, "tabla in"=w130) -> ("tabla out"=w129:string[][])  [unwired: 8 in]
        n89 = call "escribeEnTabla.vi"("parametros"=w123, "col"=w126, "tabla in"=w134) -> ("tabla out"=w135:string[][])  [unwired: 8 in]
        n90 = call "escribeEnTabla.vi"("parametros"=w123, "col"=w126, "tabla in"=w132) -> ("tabla out"=w131:string[][])  [unwired: 8 in]
        n91 = call "escribeEnTabla.vi"("parametros"=w123, "col"=w126, "tabla in"=w129) -> ("tabla out"=w136:string[][])  [unwired: 8 in]
        n92 = Bundle By Name(cluster=w142, "Tabla_A"=w135, "Tabla_C"=w131, "Tabla_Z"=w136) -> (w138:refnum<class "Prueba04.lvclass">)
        n93 = call-poly "Enqueue Message.vi"("error in (no error)"=w143, "Message"="lee_referencia", "Message Queue"=w122) -> ("error out"=w144:errorcluster)  [unwired: 7 in, 1 out]
      }
      frame "lee_referencia" {
        # "para las 3 tablas"
        # "Leer desde D28 en BD Sonometro"
        n94 = Unbundle By Name(w161) -> ("Tabla_A"=w158:string[][], "Tabla_C"=w157:string[][], "Tabla_Z"=w156:string[][], "RangoMaxRef(dB)"=w146:dbl, "Frecuencias(Hz)"=w150:string[])
        "rangoRefA_1" <- w146
        "rangoRefC_1" <- w146
        "rangoRefZ_1" <- w146
        n95 = Array Size(array=w150) -> (size(s)=w148:i32)
        n96 = Subtract(x=w146, y=45.0) -> (x-y=w145:dbl)
        "niveldBA_1" <- w145
        "niveldBC_1" <- w145
        "niveldBZ_1" <- w145
        n97 = Number To Fractional String(number=w145, precision (6)=i16 1) -> (F-format string=w149:string)  [unwired: 2 in]
        n98 = Initialize Array(w149, w148) -> (w147:string[])
        n99 = call "escribeEnTabla.vi"("parametros"=w147, "col"=2, "tabla in"=w158) -> ("tabla out"=w155:string[][])  [unwired: 8 in]
        n100 = call "escribeEnTabla.vi"("parametros"=w147, "col"=2, "tabla in"=w157) -> ("tabla out"=w154:string[][])  [unwired: 8 in]
        n101 = call "escribeEnTabla.vi"("parametros"=w147, "col"=2, "tabla in"=w156) -> ("tabla out"=w153:string[][])  [unwired: 8 in]
        n102 = Bundle By Name(cluster=w161, "Tabla_A"=w155, "Tabla_C"=w154, "Tabla_Z"=w153) -> (w162:refnum<class "Prueba04.lvclass">)
      }
      frame "Inicializar_Instrumento_A" {
        w174 = "Inicializar_Instrumento" ("Message")
        # "Inicializa todos los instrumentos"
        # "Prepara la frec y amplitusd para comenzar\nla generacion de la señal"
        n103 = local read "VoltAjuste_A"() -> (w167:T2)
        n104 = Unbundle By Name(w181) -> ("Inst_DS360"=w180:refnum<queue>, "Inst_CNT90"=w177:refnum<queue>, "Inst_Keithley2002"=w176:refnum<queue>)
        n105 = property on="cb_frec_A_1" class="CmbBox"() -> ("Value"=w184:string)  [unwired: 2 in, 2 out]
        n106 = Divide(x=w167, y=T2 1000.0) -> (x/y=w165:T2)
        n107 = Fract/Exp String To Number(string=w184) -> (number=w168:dbl)  [unwired: 3 in, 1 out]
        "frecA1" <- w168
        n108 = call-poly "Enqueue Message.vi"("error in (no error)"=w170, "Message Data"=w165, "Message"=w174, "Message Queue"=w176) -> ("error out"=w171:errorcluster)  [unwired: 6 in, 1 out]
        n109 = call-poly "Enqueue Message.vi"("error in (no error)"=w171, "Message Data"=w168, "Message"=w174, "Message Queue"=w177) -> ("error out"=w175:errorcluster)  [unwired: 6 in, 1 out]
        n110 = Bundle By Name(cluster=T5 {"frec"=0.0, "amp"=0.0, "letra"="A1"}, "frec"=w168, "amp"=w165, "letra"="A1") -> (w169:T5)
        n111 = call-poly "Enqueue Message.vi"("error in (no error)"=w175, "Message Data"=w169, "Message"="Inicializar_Instrumento", "Message Queue"=w180) -> ("error out"=w173:errorcluster)  [unwired: 6 in, 1 out]
        n112 = Bundle By Name(cluster=w183, "frec"=w168, "amp"=w165) -> (w182:refnum<class "Prueba04.lvclass">)
      }
      frame "Inicializar_Instrumento_C" {
        w194 = "Inicializar_Instrumento" ("Message")
        # "Inicializa todos los instrumentos"
        # "Prepara la frec y amplitusd para comenzar\nla generacion de la señal"
        n113 = local read "VoltAjuste_C"() -> (w187:T2)
        n114 = Unbundle By Name(w201) -> ("Inst_DS360"=w200:refnum<queue>, "Inst_CNT90"=w197:refnum<queue>, "Inst_Keithley2002"=w196:refnum<queue>)
        n115 = property on="cb_frec_C_1" class="CmbBox"() -> ("Value"=w204:string)  [unwired: 2 in, 2 out]
        n116 = Divide(x=w187, y=T2 1000.0) -> (x/y=w185:T2)
        n117 = Fract/Exp String To Number(string=w204) -> (number=w188:dbl)  [unwired: 3 in, 1 out]
        "frecC1" <- w188
        n118 = call-poly "Enqueue Message.vi"("error in (no error)"=w190, "Message Data"=w185, "Message"=w194, "Message Queue"=w196) -> ("error out"=w191:errorcluster)  [unwired: 6 in, 1 out]
        n119 = call-poly "Enqueue Message.vi"("error in (no error)"=w191, "Message Data"=w188, "Message"=w194, "Message Queue"=w197) -> ("error out"=w195:errorcluster)  [unwired: 6 in, 1 out]
        n120 = Bundle By Name(cluster=T5 {"frec"=0.0, "amp"=0.0, "letra"="A1"}, "frec"=w188, "amp"=w185, "letra"="A1") -> (w189:T5)
        n121 = call-poly "Enqueue Message.vi"("error in (no error)"=w195, "Message Data"=w189, "Message"="Inicializar_Instrumento", "Message Queue"=w200) -> ("error out"=w193:errorcluster)  [unwired: 6 in, 1 out]
        n122 = Bundle By Name(cluster=w203, "frec"=w188, "amp"=w185) -> (w202:refnum<class "Prueba04.lvclass">)
      }
      frame "Inicializar_Instrumento_Z" {
        w214 = "Inicializar_Instrumento" ("Message")
        # "Inicializa todos los instrumentos"
        # "Prepara la frec y amplitusd para comenzar\nla generacion de la señal"
        n123 = Unbundle By Name(w221) -> ("Inst_DS360"=w220:refnum<queue>, "Inst_CNT90"=w217:refnum<queue>, "Inst_Keithley2002"=w216:refnum<queue>)
        n124 = local read "VoltAjuste_Z"() -> (w207:T2)
        n125 = property on="cb_frec_Z_1" class="CmbBox"() -> ("Value"=w224:string)  [unwired: 2 in, 2 out]
        n126 = Divide(x=w207, y=T2 1000.0) -> (x/y=w205:T2)
        n127 = Fract/Exp String To Number(string=w224) -> (number=w208:dbl)  [unwired: 3 in, 1 out]
        "frecZ1" <- w208
        n128 = call-poly "Enqueue Message.vi"("error in (no error)"=w210, "Message Data"=w205, "Message"=w214, "Message Queue"=w216) -> ("error out"=w211:errorcluster)  [unwired: 6 in, 1 out]
        n129 = call-poly "Enqueue Message.vi"("error in (no error)"=w211, "Message Data"=w208, "Message"=w214, "Message Queue"=w217) -> ("error out"=w215:errorcluster)  [unwired: 6 in, 1 out]
        n130 = Bundle By Name(cluster=T5 {"frec"=0.0, "amp"=0.0, "letra"="A1"}, "frec"=w208, "amp"=w205, "letra"="A1") -> (w209:T5)
        n131 = call-poly "Enqueue Message.vi"("error in (no error)"=w215, "Message Data"=w209, "Message"="Inicializar_Instrumento", "Message Queue"=w220) -> ("error out"=w213:errorcluster)  [unwired: 6 in, 1 out]
        n132 = Bundle By Name(cluster=w223, "frec"=w208, "amp"=w205) -> (w222:refnum<class "Prueba04.lvclass">)
      }
      frame "Detener_Instrumento" {
        w225 = "Detener_Instrumento" ("Message")
        # "Detiene todos los instrumentos"
        n133 = Unbundle By Name(w231) -> ("Inst_DS360"=w230:refnum<queue>, "Inst_CNT90"=w229:refnum<queue>, "Inst_Keithley2002"=w228:refnum<queue>)
        n134 = call-poly "Enqueue Message.vi"("error in (no error)"=w234, "Message"=w225, "Message Queue"=w228) -> ("error out"=w227:errorcluster)  [unwired: 7 in, 1 out]
        n135 = call-poly "Enqueue Message.vi"("error in (no error)"=w227, "Message"=w225, "Message Queue"=w229) -> ("error out"=w226:errorcluster)  [unwired: 7 in, 1 out]
        n136 = call-poly "Enqueue Message.vi"("error in (no error)"=w226, "Message"=w225, "Message Queue"=w230) -> ("error out"=w232:errorcluster)  [unwired: 7 in, 1 out]
      }
      frame "guardarVrefA" {
        n137 = flat-sequence {
          tunnel: w238 -> [w243]
          tunnel: [w243] -> w236
          frame #0 {
            n138 = local read "VoltAjuste_A"() -> (w240:T2)
            n139 = Divide(x=w240, y=T2 1000.0) -> (x/y=→"Vref_A":T2)
            n140 = Number To Fractional String(number=w240, precision (6)=i16 1) -> (F-format string=w247:string)  [unwired: 2 in]
            n141 = Format Into String(format string="Se guardó Vref = %s mV", w247) -> (resulting string=w244:string)  [unwired: 2 in, 1 out]
            n142 = One Button Dialog(message=w244) -> ()  [unwired: 1 in, 1 out]
          }
        }
        n143 = property on="ir a resultados_A" class="Bool"(error in=w236, "DisabledEnum"=T3."Enabled" ("Disabled")) -> (error out=w235:errorcluster)  [unwired: 1 in, 1 out]
      }
      frame "guardarVrefC" {
        n144 = flat-sequence {
          tunnel: w251 -> [w256]
          tunnel: [w256] -> w249
          frame #0 {
            n145 = local read "VoltAjuste_C"() -> (w254:T2)
            n146 = Divide(x=w254, y=T2 1000.0) -> (x/y=→"Vref_C":T2)
            n147 = Number To Fractional String(number=w254, precision (6)=i16 1) -> (F-format string=w260:string)  [unwired: 2 in]
            n148 = Format Into String(format string="Se guardó Vref = %s mV", w260) -> (resulting string=w257:string)  [unwired: 2 in, 1 out]
            n149 = One Button Dialog(message=w257) -> ()  [unwired: 1 in, 1 out]
          }
        }
        n150 = property on="ir a resultados_C" class="Bool"(error in=w249, "DisabledEnum"=T3."Enabled" ("Disabled")) -> (error out=w248:errorcluster)  [unwired: 1 in, 1 out]
      }
      frame "guardarVrefZ" {
        n151 = flat-sequence {
          tunnel: w264 -> [w269]
          tunnel: [w269] -> w262
          frame #0 {
            n152 = local read "VoltAjuste_Z"() -> (w267:T2)
            n153 = Divide(x=w267, y=T2 1000.0) -> (x/y=→"Vref_Z":T2)
            n154 = Number To Fractional String(number=w267, precision (6)=i16 1) -> (F-format string=w273:string)  [unwired: 2 in]
            n155 = Format Into String(format string="Se guardó Vref = %s mV", w273) -> (resulting string=w270:string)  [unwired: 2 in, 1 out]
            n156 = One Button Dialog(message=w270) -> ()  [unwired: 1 in, 1 out]
          }
        }
        n157 = property on="ir a resultados _Z" class="Bool"(error in=w262, "DisabledEnum"=T3."Enabled" ("Disabled")) -> (error out=w261:errorcluster)  [unwired: 1 in, 1 out]
      }
      frame "iniciarGEN_A1" {
        n158 = Unbundle By Name(w276) -> ("Inst_DS360"=w282:refnum<queue>)
        n159 = call-poly "Enqueue Message.vi"("error in (no error)"=w277, "Message"="Habilitar_Generador", "Message Queue"=w282) -> ("error out"=w280:errorcluster)  [unwired: 7 in, 1 out]
        n160 = call "Time Delay3"("error in (no error)"=w280, "Delay Time (s)"=0.5) -> ("error out"=w279:errorcluster)  [unwired: 9 in]
        n161 = call-poly "Enqueue Message.vi"("error in (no error)"=w279, "Message"="Leer_Voltaje", "Message Queue"=w274) -> ("error out"=w275:errorcluster)  [unwired: 7 in, 1 out]
      }
      frame "iniciarGEN_C1" {
        n162 = Unbundle By Name(w287) -> ("Inst_DS360"=w293:refnum<queue>)
        n163 = call-poly "Enqueue Message.vi"("error in (no error)"=w288, "Message"="Habilitar_Generador", "Message Queue"=w293) -> ("error out"=w291:errorcluster)  [unwired: 7 in, 1 out]
        n164 = call "Time Delay7"("error in (no error)"=w291, "Delay Time (s)"=0.5) -> ("error out"=w290:errorcluster)  [unwired: 9 in]
        n165 = call-poly "Enqueue Message.vi"("error in (no error)"=w290, "Message"="Leer_Voltaje", "Message Queue"=w285) -> ("error out"=w286:errorcluster)  [unwired: 7 in, 1 out]
      }
      frame "iniciarGEN_Z1" {
        n166 = Unbundle By Name(w298) -> ("Inst_DS360"=w304:refnum<queue>)
        n167 = call-poly "Enqueue Message.vi"("error in (no error)"=w299, "Message"="Habilitar_Generador", "Message Queue"=w304) -> ("error out"=w302:errorcluster)  [unwired: 7 in, 1 out]
        n168 = call "Time Delay8"("error in (no error)"=w302, "Delay Time (s)"=0.5) -> ("error out"=w301:errorcluster)  [unwired: 9 in]
        n169 = call-poly "Enqueue Message.vi"("error in (no error)"=w301, "Message"="Leer_Voltaje", "Message Queue"=w296) -> ("error out"=w297:errorcluster)  [unwired: 7 in, 1 out]
      }
      frame "ConfigurarGEN_A2" {
        # "volt"
        # "frec"
        # "cambia el valor del Combo Box"
        # "obtengo \nfrecuencia a generar"
        n170 = Flush Queue(queue=w323, error in (no error)=w329) -> (error out=w315:errorcluster)  [unwired: 2 out]
        n171 = call "FGV_fila.vi"("action"=enum16{"increment", "set_start", "get"}."get") -> ("fila out"=w331:i32)  [unwired: 3 in, 1 out]
        "fila actual A" <- w331
        n172 = Unbundle By Name(w327) -> ("Tabla_A"=w326:string[][])
        n173 = Index Array(array=w326, index (row) #1=w331, index (col) #1=0 ("disabled index (col)"), index (row) #2=w331, index (col) #2=1 ("disabled index (col)")) -> (element #1=w325:string, element #2=w324:string)
        "frec_generar_A2" <- w325
        "volt_generar_A2" <- w324
        n174 = Unbundle By Name(w321) -> ("Inst_DS360"=w320:refnum<queue>, "Inst_Keithley2002"=w311:refnum<queue>, "Inst_CNT90"=w312:refnum<queue>)
        n175 = property on="cb_frec_A_2" class="CmbBox"() -> ("Strings[]"=w334:string[])  [unwired: 2 in, 2 out]
        n176 = Fract/Exp String To Number(string=w324) -> (number=w308:dbl)  [unwired: 3 in, 1 out]
        n177 = Fract/Exp String To Number(string=w325) -> (number=w307:dbl)  [unwired: 3 in, 1 out]
        n178 = Index Array(array=w334, index=w331) -> (element=w333:string)
        n179 = property on="cb_frec_A_2" class="CmbBox"("Value"=w333) -> ()  [unwired: 2 in, 2 out]
        n180 = call-poly "Enqueue Message.vi"("error in (no error)"=w315, "Message Data"=w307, "Message"="EnviarFrecuenciaRef", "Message Queue"=w312) -> ("error out"=w314:errorcluster)  [unwired: 6 in, 1 out]
        n181 = Bundle By Name(cluster=w327, "frec"=w307, "amp"=w308) -> (w328:refnum<class "Prueba04.lvclass">)
        n182 = call-poly "Enqueue Message.vi"("error in (no error)"=w314, "Message Data"=w308, "Message"="ActualizarVoltaje", "Message Queue"=w311) -> ("error out"=w313:errorcluster)  [unwired: 6 in, 1 out]
        n183 = Bundle By Name(cluster=T5 {"frec"=0.0, "amp"=0.0, "letra"="A1"} ("setpoint"), "frec"=w307, "amp"=w308, "letra"="A2" ("message")) -> (w318:T5)
        n184 = call-poly "Enqueue Message.vi"("error in (no error)"=w313, "Message Data"=w318, "Message"="ActualizarHz&Amp", "Message Queue"=w320) -> ("error out"=w322:errorcluster)  [unwired: 6 in, 1 out]
      }
      frame "ConfigurarGEN_C2" {
        # "volt"
        # "frec"
        # "cambia el valor del Combo Box"
        # "obtengo \nfrecuencia a generar"
        n185 = Flush Queue(queue=w349, error in (no error)=w356) -> (error out=w355:errorcluster)  [unwired: 2 out]
        n186 = call "FGV_fila.vi"("action"=enum16{"increment", "set_start", "get"}."get") -> ("fila out"=w358:i32)  [unwired: 3 in, 1 out]
        "fila actual C" <- w358
        n187 = Unbundle By Name(w353) -> ("Tabla_C"=w352:string[][])
        n188 = Index Array(array=w352, index (row) #1=w358, index (col) #1=0 ("disabled index (col)"), index (row) #2=w358, index (col) #2=1 ("disabled index (col)")) -> (element #1=w351:string, element #2=w350:string)
        "frec_generar_C2" <- w351
        "volt_generar_C2" <- w350
        n189 = property on="cb_frec_C_2" class="CmbBox"() -> ("Strings[]"=w361:string[])  [unwired: 2 in, 2 out]
        n190 = Index Array(array=w361, index=w358) -> (element=w360:string)
        n191 = Unbundle By Name(w347) -> ("Inst_DS360"=w344:refnum<queue>, "Inst_CNT90"=w345:refnum<queue>, "Inst_Keithley2002"=w346:refnum<queue>)
        n192 = Fract/Exp String To Number(string=w350) -> (number=w339:dbl)  [unwired: 3 in, 1 out]
        n193 = Fract/Exp String To Number(string=w351) -> (number=w340:dbl)  [unwired: 3 in, 1 out]
        n194 = property on="cb_frec_C_2" class="CmbBox"("Value"=w360) -> ()  [unwired: 2 in, 2 out]
        n195 = call-poly "Enqueue Message.vi"("Message Data"=w339, "Message"="ActualizarVoltaje", "Message Queue"=w346) -> ()  [unwired: 7 in, 2 out]
        n196 = call-poly "Enqueue Message.vi"("Message Data"=w340, "Message"="EnviarFrecuenciaRef", "Message Queue"=w345) -> ()  [unwired: 7 in, 2 out]
        n197 = Bundle By Name(cluster=w353, "frec"=w340, "amp"=w339) -> (w354:refnum<class "Prueba04.lvclass">)
        n198 = Bundle By Name(cluster=T5 {"frec"=0.0, "amp"=0.0, "letra"="A1"} ("setpoint"), "frec"=w340, "amp"=w339, "letra"="C2" ("Message")) -> (w342:T5)
        n199 = call-poly "Enqueue Message.vi"("error in (no error)"=w355, "Message Data"=w342, "Message"="ActualizarHz&Amp", "Message Queue"=w344) -> ("error out"=w348:errorcluster)  [unwired: 6 in, 1 out]
      }
      frame "ConfigurarGEN_Z2" {
        # "volt"
        # "frec"
        # "cambia el valor del Combo Box"
        # "obtengo \nfrecuencia a generar"
        n200 = Flush Queue(queue=w379, error in (no error)=w385) -> (error out=w378:errorcluster)  [unwired: 2 out]
        n201 = call "FGV_fila.vi"("action"=enum16{"increment", "set_start", "get"}."get") -> ("fila out"=w387:i32)  [unwired: 3 in, 1 out]
        "fila actual Z" <- w387
        n202 = Unbundle By Name(w383) -> ("Tabla_Z"=w382:string[][])
        n203 = Index Array(array=w382, index (row) #1=w387, index (col) #1=0 ("disabled index (col)"), index (row) #2=w387, index (col) #2=1 ("disabled index (col)")) -> (element #1=w381:string, element #2=w380:string)
        "frec_generar_Z2" <- w381
        "volt_generar_Z2" <- w380
        n204 = property on="cb_frec_Z_2" class="CmbBox"() -> ("Strings[]"=w390:string[])  [unwired: 2 in, 2 out]
        n205 = Unbundle By Name(w374) -> ("Inst_DS360"=w371:refnum<queue>, "Inst_CNT90"=w372:refnum<queue>, "Inst_Keithley2002"=w373:refnum<queue>)
        n206 = Fract/Exp String To Number(string=w380) -> (number=w366:dbl)  [unwired: 3 in, 1 out]
        n207 = Fract/Exp String To Number(string=w381) -> (number=w367:dbl)  [unwired: 3 in, 1 out]
        n208 = Index Array(array=w390, index=w387) -> (element=w389:string)
        n209 = property on="cb_frec_Z_2" class="CmbBox"("Value"=w389) -> ()  [unwired: 2 in, 2 out]
        n210 = call-poly "Enqueue Message.vi"("error in (no error)"=w378, "Message Data"=w366, "Message"="ActualizarVoltaje", "Message Queue"=w373) -> ("error out"=w377:errorcluster)  [unwired: 6 in, 1 out]
        n211 = Bundle By Name(cluster=w383, "frec"=w367, "amp"=w366) -> (w384:refnum<class "Prueba04.lvclass">)
        n212 = call-poly "Enqueue Message.vi"("error in (no error)"=w377, "Message Data"=w367, "Message"="EnviarFrecuenciaRef", "Message Queue"=w372) -> ("error out"=w376:errorcluster)  [unwired: 6 in, 1 out]
        n213 = Bundle By Name(cluster=T5 {"frec"=0.0, "amp"=0.0, "letra"="A1"} ("setpoint"), "frec"=w367, "amp"=w366, "letra"="Z2" ("Message")) -> (w368:T5)
        n214 = call-poly "Enqueue Message.vi"("error in (no error)"=w376, "Message Data"=w368, "Message"="ActualizarHz&Amp", "Message Queue"=w371) -> ("error out"=w375:errorcluster)  [unwired: 6 in, 1 out]
      }
      frame "iniciarGEN_A2" {
        n215 = Unbundle By Name(w395) -> ("Inst_DS360"=w401:refnum<queue>)
        n216 = call-poly "Enqueue Message.vi"("error in (no error)"=w396, "Message"="Habilitar_Generador", "Message Queue"=w401) -> ("error out"=w399:errorcluster)  [unwired: 7 in, 1 out]
        n217 = call "Time Delay10"("error in (no error)"=w399, "Delay Time (s)"=0.5) -> ("error out"=w398:errorcluster)  [unwired: 9 in]
        n218 = local write "generarA2"(TRUE ("generarA_1")) -> ()
        n219 = call-poly "Enqueue Message.vi"("error in (no error)"=w398, "Message"="Leer_Voltaje", "Message Queue"=w394) -> ("error out"=w393:errorcluster)  [unwired: 7 in, 1 out]
      }
      frame "iniciarGEN_C2" {
        n220 = Unbundle By Name(w407) -> ("Inst_DS360"=w413:refnum<queue>)
        n221 = call-poly "Enqueue Message.vi"("error in (no error)"=w408, "Message"="Habilitar_Generador", "Message Queue"=w413) -> ("error out"=w411:errorcluster)  [unwired: 7 in, 1 out]
        n222 = call "Time Delay11"("error in (no error)"=w411, "Delay Time (s)"=0.5) -> ("error out"=w410:errorcluster)  [unwired: 9 in]
        n223 = local write "generarC2"(TRUE ("generarA_1")) -> ()
        n224 = call-poly "Enqueue Message.vi"("error in (no error)"=w410, "Message"="Leer_Voltaje", "Message Queue"=w406) -> ("error out"=w405:errorcluster)  [unwired: 7 in, 1 out]
      }
      frame "iniciarGEN_Z2" {
        n225 = Unbundle By Name(w419) -> ("Inst_DS360"=w425:refnum<queue>)
        n226 = call-poly "Enqueue Message.vi"("error in (no error)"=w420, "Message"="Habilitar_Generador", "Message Queue"=w425) -> ("error out"=w423:errorcluster)  [unwired: 7 in, 1 out]
        n227 = local write "generarZ2"(TRUE ("generarA_1")) -> ()
        n228 = call "Time Delay12"("error in (no error)"=w423, "Delay Time (s)"=0.5) -> ("error out"=w422:errorcluster)  [unwired: 9 in]
        n229 = call-poly "Enqueue Message.vi"("error in (no error)"=w422, "Message"="Leer_Voltaje", "Message Queue"=w418) -> ("error out"=w417:errorcluster)  [unwired: 7 in, 1 out]
      }
      frame "Leer_Voltaje" {
        n230 = Flush Queue(queue=w430, error in (no error)=w431) -> (queue out=w432:refnum<queue>, error out=w433:errorcluster)  [unwired: 1 out]
        n231 = Unbundle By Name(w429) -> ("Inst_Keithley2002"=w436:refnum<queue>)
        n232 = call-poly "Enqueue Message.vi"("error in (no error)"=w433, "Message"="Leer_Frecuencia", "Message Queue"=w432) -> ("error out"=w439:errorcluster)  [unwired: 7 in, 1 out]
        n233 = call-poly "Enqueue Message.vi"("error in (no error)"=w439, "Message"="Leer_Instrumento", "Message Queue"=w436) -> ("error out"=w437:errorcluster)  [unwired: 7 in, 1 out]
        n234 = call "Time Delay"("error in (no error)"=w437, "Delay Time (s)"=1.0) -> ("error out"=w428:errorcluster)  [unwired: 9 in]
      }
      frame "Leer_Frecuencia" {
        n235 = Flush Queue(queue=w443, error in (no error)=w444) -> (queue out=w445:refnum<queue>, error out=w446:errorcluster)  [unwired: 1 out]
        n236 = Unbundle By Name(w442) -> ("Inst_CNT90"=w449:refnum<queue>)
        n237 = call-poly "Enqueue Message.vi"("error in (no error)"=w446, "Message"="Leer_Indicadores", "Message Queue"=w445) -> ("error out"=w452:errorcluster)  [unwired: 7 in, 1 out]
        n238 = call-poly "Enqueue Message.vi"("error in (no error)"=w452, "Message"="Leer_Instrumento", "Message Queue"=w449) -> ("error out"=w450:errorcluster)  [unwired: 7 in, 1 out]
        n239 = call "Time Delay2"("error in (no error)"=w450, "Delay Time (s)"=1.0) -> ("error out"=w441:errorcluster)  [unwired: 9 in]
      }
      frame "Leer_Indicadores" {
        n240 = Flush Queue(queue=w460, error in (no error)=w461) -> (queue out=w462:refnum<queue>, error out=w463:errorcluster)  [unwired: 1 out]
        n241 = Unbundle By Name(w458) -> ("frecMonA_1"=w457:refnum<vi>, "voltMonA_1"=w455:refnum<vi>)
        n242 = call-poly "Enqueue Message.vi"("error in (no error)"=w463, "Message"="Leer_Voltaje", "Message Queue"=w462) -> ("error out"=w466:errorcluster)  [unwired: 7 in, 1 out]
        n243 = property class="DigNum (strict)"(reference=w457) -> ("Value"=→"frecMonA_2" →"frecMonC_1" →"frecMonC_2" →"frecMonZ_2" →"frecMonZ_1":dbl)  [unwired: 1 in, 2 out]
        n244 = property class="DigNum (strict)"(reference=w455) -> ("Value"=→"voltMonZ_2" →"voltMonA_2" →"voltMonC_1" →"voltMonC_2" →"voltMonZ_1":dbl)  [unwired: 1 in, 2 out]
        n245 = call "Time Delay4"("error in (no error)"=w466, "Delay Time (s)"=1.0) -> ("error out"=w459:errorcluster)  [unwired: 9 in]
      }
      frame "EnviarVoltajeGEN" {
        n246 = Unbundle By Name(w469) -> ("Inst_DS360"=w477:refnum<queue>, "Inst_Keithley2002"=w482:refnum<queue>)
        n247 = Variant To Data(error in=w470, type=0.0, Variant=w467) -> (data=w475:dbl, error out=w480:errorcluster)
        n248 = call "Time Delay6"("error in (no error)"=w480, "Delay Time (s)"=0.5) -> ("error out"=w472:errorcluster)  [unwired: 9 in]
        n249 = call-poly "Enqueue Message.vi"("error in (no error)"=w472, "Message Data"=w475, "Message"="ActualizarVoltaje", "Message Queue"=w482) -> ("error out"=w478:errorcluster)  [unwired: 6 in, 1 out]
        n250 = call "Time Delay5"("error in (no error)"=w478, "Delay Time (s)"=0.5) -> ("error out"=w474:errorcluster)  [unwired: 9 in]
        n251 = call-poly "Enqueue Message.vi"("error in (no error)"=w474, "Message Data"=w475, "Message"="ActualizarAmplitud", "Message Queue"=w477) -> ("error out"=w468:errorcluster)  [unwired: 6 in, 1 out]
      }
      frame "detenerGEN" {
        w497 = 0.0 ("frecMonA_1")
        w498 = 0.0 ("frecMonA_1")
        n252 = Unbundle By Name(w485) -> ("Inst_DS360"=w489:refnum<queue>)
        n253 = call "Time Delay9"("error in (no error)"=w486, "Delay Time (s)"=0.5) -> ("error out"=w487:errorcluster)  [unwired: 9 in]
        n254 = local write "frecMonA_1"(w498) -> ()
        n255 = local write "voltMonA_1"(w498) -> ()
        n256 = local write "voltMonA_2"(w498) -> ()
        n257 = local write "frecMonA_2"(w498) -> ()
        n258 = local write "voltMonC_1"(w498) -> ()
        n259 = local write "frecMonC_1"(w498) -> ()
        n260 = call-poly "Enqueue Message.vi"("error in (no error)"=w487, "Message"="Deshabilitar_Generador", "Message Queue"=w489) -> ("error out"=w484:errorcluster)  [unwired: 7 in, 1 out]
        n261 = local write "voltMonC_2"(w497) -> ()
        n262 = local write "frecMonC_2"(w497) -> ()
        n263 = local write "voltMonZ_1"(w497) -> ()
        n264 = local write "frecMonZ_1"(w497) -> ()
        n265 = local write "voltMonZ_2"(w497) -> ()
        n266 = local write "frecMonZ_2"(w497) -> ()
        n267 = Unbundle By Name(w493) -> ("Control references"=w492:T6)
        n268 = call-poly "get control reference by name.vi"("error in (no error)"=w484, "Control names"=string[] ["guardar_Vref_A", "guardar_Vref_C", "guardar_Vref_Z", "guardar_Vref_A", "guardar_Vref_C", "guardar_Vref_Z"] ("Control name"), "Control references"=w492) -> ("error out"=w494:errorcluster, "References"=w496:refnum<vi>[])  [unwired: 3 in]
        n269 = call "Enable_Visible Buttons.vi"("Enable? (T)"=FALSE, "Controls Ref Array"=w496) -> ()  [unwired: 10 in]
      }
      frame "crea_voltajes_prueba_A" {
        # "Vf1 =(VRef) x 10 ^( Pf1 / 20)\n\nVf1 = Voltaje para frecuencia 1\nVref = Voltaje de referencia según ajuste\nPf1= Ponderación A según Base de datos"
        n270 = property on="cb_frec_A_2" class="CmbBox"() -> ("Value"=→"frec_ref_A":string)  [unwired: 2 in, 2 out]
        n271 = Unbundle By Name(w503) -> ("Ponderaciones A"=w502:dbl[])
        n272 = call-poly "Enqueue Message.vi"("error in (no error)"=w507, "Message"="voltajeInicialA2", "Message Queue"=w501) -> ("error out"=w500:errorcluster)  [unwired: 7 in, 1 out]
        n273 = for {
          tunnel: [w514] -> w509 mode=indexing
          tunnel: w502 -> [w511] mode=indexing
          # "V"
          # "mV"
          # "Volts"
          # "Pfx"
          n274 = local read "Vref_A"() -> (w513:dbl)
          n275 = Divide(x=w511, y=20.0) -> (x/y=w517:dbl)
          n276 = Power Of X(1:10.0 ("x"), 2:w517) -> (0:w516:dbl)
          n277 = Multiply(x=w516, y=w513) -> (x*y=w512:dbl)
          n278 = Number To Fractional String(number=w512, precision (6)=i16 3) -> (F-format string=w514:string)  [unwired: 2 in]
        }
        "Voltajes_Ref_A" <- w509
        n279 = Unbundle By Name(w503) -> ("Tabla_A"=w506:string[][])
        n280 = call "escribeEnTabla.vi"("parametros"=w509, "col"=1, "tabla in"=w506) -> ("tabla out"=w504:string[][])  [unwired: 8 in]
        n281 = Bundle By Name(cluster=w503, "Tabla_A"=w504) -> (w505:refnum<class "Prueba04.lvclass">)
        n282 = local write "Tabla_A"(w504) -> ()
      }
      frame "crea_voltajes_prueba_C" {
        # "Vf1 =(VRef) x 10 ^( Pf1 / 20)\n\nVf1 = Voltaje para frecuencia 1\nVref = Voltaje de referencia según ajuste\nPf1= Ponderación A según Base de datos"
        n283 = property on="cb_frec_C_2" class="CmbBox"() -> ("Value"=→"frec_ref_C":string)  [unwired: 2 in, 2 out]
        n284 = Flush Queue(queue=w523, error in (no error)=w531) -> (queue out=w521:refnum<queue>, error out=w530:errorcluster)  [unwired: 1 out]
        n285 = Unbundle By Name(w525) -> ("Ponderaciones C"=w524:dbl[])
        n286 = call-poly "Enqueue Message.vi"("error in (no error)"=w530, "Message"="voltajeInicialC2", "Message Queue"=w521) -> ("error out"=w522:errorcluster)  [unwired: 7 in, 1 out]
        n287 = for {
          tunnel: w524 -> [w542] mode=indexing
          tunnel: [w534] -> w529 mode=indexing
          # "Pfx"
          n288 = local read "Vref_C"() -> (w537:dbl)
          n289 = Divide(x=w542, y=20.0) -> (x/y=w539:dbl)
          n290 = Power Of X(1:10.0 ("x"), 2:w539) -> (0:w538:dbl)
          n291 = Multiply(x=w538, y=w537) -> (x*y=w536:dbl)
          n292 = Number To Fractional String(number=w536, precision (6)=i16 3) -> (F-format string=w534:string)  [unwired: 2 in]
        }
        "Voltajes_Ref_C" <- w529
        n293 = Unbundle By Name(w525) -> ("Tabla_C"=w528:string[][])
        n294 = call "escribeEnTabla.vi"("parametros"=w529, "col"=1, "tabla in"=w528) -> ("tabla out"=w526:string[][])  [unwired: 8 in]
        n295 = Bundle By Name(cluster=w525, "Tabla_C"=w526) -> (w527:refnum<class "Prueba04.lvclass">)
        n296 = local write "Tabla_C"(w526) -> ()
      }
      frame "crea_voltajes_prueba_Z" {
        # "Vf1 =(VRef) x 10 ^( Pf1 / 20)\n\nVf1 = Voltaje para frecuencia 1\nVref = Voltaje de referencia según ajuste\nPf1= Ponderación A según Base de datos"
        n297 = Flush Queue(queue=w546, error in (no error)=w554) -> (queue out=w544:refnum<queue>, error out=w553:errorcluster)  [unwired: 1 out]
        n298 = property on="cb_frec_Z_2" class="CmbBox"() -> ("Value"=→"frec_ref_Z_2":string)  [unwired: 2 in, 2 out]
        n299 = Unbundle By Name(w548) -> ("Ponderaciones Z"=w547:dbl[])
        n300 = call-poly "Enqueue Message.vi"("error in (no error)"=w553, "Message"="voltajeInicialZ2", "Message Queue"=w544) -> ("error out"=w545:errorcluster)  [unwired: 7 in, 1 out]
        n301 = for {
          tunnel: [w558] -> w552 mode=indexing
          tunnel: w547 -> [w557] mode=indexing
          # "Pfx"
          n302 = local read "Vref_Z"() -> (w561:dbl)
          n303 = Divide(x=w557, y=20.0) -> (x/y=w563:dbl)
          n304 = Power Of X(1:10.0 ("x"), 2:w563) -> (0:w562:dbl)
          n305 = Multiply(x=w562, y=w561) -> (x*y=w560:dbl)
          n306 = Number To Fractional String(number=w560, precision (6)=i16 3) -> (F-format string=w558:string)  [unwired: 2 in]
        }
        "Voltajes_Ref_Z" <- w552
        n307 = Unbundle By Name(w548) -> ("Tabla_Z"=w551:string[][])
        n308 = call "escribeEnTabla.vi"("parametros"=w552, "col"=1, "tabla in"=w551) -> ("tabla out"=w549:string[][])  [unwired: 8 in]
        n309 = local write "Tabla_Z"(w549) -> ()
        n310 = Bundle By Name(cluster=w548, "Tabla_Z"=w549) -> (w550:refnum<class "Prueba04.lvclass">)
      }
      frame "voltajeInicialA2" {
        n311 = call-poly "Enqueue Message.vi"("error in (no error)"=w570, "Message"="ConfigurarGEN_A2", "Message Queue"=w567) -> ("error out"=w568:errorcluster)  [unwired: 7 in, 1 out]
        n312 = local read "Voltajes_Ref_A"() -> (w572:string[])
        n313 = call "FGV_fila.vi"("action"=enum16{"increment", "set_start", "get"}."get") -> ("fila out"=w573:i32)  [unwired: 3 in, 1 out]
        n314 = Index Array(array=w572, index=w573) -> (element=w574:string)
        n315 = Fract/Exp String To Number(string=w574) -> (number=→"voltaje_A":dbl)  [unwired: 3 in, 1 out]
      }
      frame "voltajeInicialC2" {
        n316 = call-poly "Enqueue Message.vi"("error in (no error)"=w581, "Message"="ConfigurarGEN_C2", "Message Queue"=w577) -> ("error out"=w578:errorcluster)  [unwired: 7 in, 1 out]
        n317 = local read "Voltajes_Ref_C"() -> (w583:string[])
        n318 = call "FGV_fila.vi"("action"=enum16{"increment", "set_start", "get"}."get") -> ("fila out"=w584:i32)  [unwired: 3 in, 1 out]
        n319 = Index Array(array=w583, index=w584) -> (element=w585:string)
        n320 = Fract/Exp String To Number(string=w585) -> (number=→"voltaje_C":dbl)  [unwired: 3 in, 1 out]
      }
      frame "voltajeInicialZ2" {
        n321 = call-poly "Enqueue Message.vi"("error in (no error)"=w591, "Message"="ConfigurarGEN_Z2", "Message Queue"=w587) -> ("error out"=w588:errorcluster)  [unwired: 7 in, 1 out]
        n322 = local read "Voltajes_Ref_Z"() -> (w594:string[])
        n323 = call "FGV_fila.vi"("error in (no error)"=w588, "action"=enum16{"increment", "set_start", "get"}."get") -> ("error out"=w590:errorcluster, "fila out"=w595:i32)  [unwired: 2 in]
        n324 = Index Array(array=w594, index=w595) -> (element=w596:string)
        n325 = Fract/Exp String To Number(string=w596) -> (number=→"voltaje_Z":dbl)  [unwired: 3 in, 1 out]
      }
      frame "actualizarVrefA" {
        n326 = local read "Voltajes_Ref_A"() -> (w604:string[])
        n327 = call "FGV_fila.vi"("error in (no error)"=w603, "action"=enum16{"increment", "set_start", "get"}."get") -> ("error out"=w602:errorcluster, "fila out"=w601:i32)  [unwired: 2 in]
        n328 = Index Array(array=w604, index=w601) -> (element=w600:string)
        n329 = Fract/Exp String To Number(string=w600, default (0 dbl)=0.0 ("default (0 I32)")) -> (number=w599:dbl)  [unwired: 2 in, 1 out]
        n330 = local write "voltaje_A"(w599) -> ()
      }
      frame "actualizarVrefC" {
        n331 = local read "Voltajes_Ref_C"() -> (w613:string[])
        n332 = call "FGV_fila.vi"("error in (no error)"=w612, "action"=enum16{"increment", "set_start", "get"}."get") -> ("error out"=w611:errorcluster, "fila out"=w610:i32)  [unwired: 2 in]
        n333 = Index Array(array=w613, index=w610) -> (element=w609:string)
        n334 = Fract/Exp String To Number(string=w609, default (0 dbl)=0.0 ("default (0 I32)")) -> (number=w608:dbl)  [unwired: 2 in, 1 out]
        n335 = local write "voltaje_C"(w608) -> ()
      }
      frame "actualizarVrefZ" {
        n336 = local read "Voltajes_Ref_Z"() -> (w622:string[])
        n337 = call "FGV_fila.vi"("error in (no error)"=w621, "action"=enum16{"increment", "set_start", "get"}."get") -> ("error out"=w620:errorcluster, "fila out"=w619:i32)  [unwired: 2 in]
        n338 = Index Array(array=w622, index=w619) -> (element=w618:string)
        n339 = Fract/Exp String To Number(string=w618, default (0 dbl)=0.0 ("default (0 I32)")) -> (number=w617:dbl)  [unwired: 2 in, 1 out]
        n340 = local write "voltaje_Z"(w617) -> ()
      }
      frame "ingresaMedicionesA" {
        n341 = Flush Queue(queue=w629, error in (no error)=w637) -> (queue out=w626:refnum<queue>, error out=w636:errorcluster)  [unwired: 1 out]
        n342 = Variant To Data(error in=w636, type=string[][] [] ("NewVal"), Variant=w628) -> (data=w639:string[][], error out=w641:errorcluster)
        n343 = Unbundle By Name(w635) -> ("Tabla_A"=w634:string[][], "mediciones"=w631:T7)
        n344 = control-ref of="Tabla_A"() -> (w638:refnum<vi>)
        n345 = call "ingresaMediciones.vi"("New Value"=w639, "Tbl Refnum"=w638, "error in (no error)"=w641, "mediciones in"=w631, "Tabla in"=w634) -> ("error out"=w640:errorcluster, "mediciones out"=w630:T7, "Tabla out"=w632:string[][])  [unwired: 3 in, 1 out]
        n346 = Bundle By Name(cluster=w635, "Tabla_A"=w632, "mediciones"=w630) -> (w633:refnum<class "Prueba04.lvclass">)
        n347 = call-poly "Enqueue Message.vi"("error in (no error)"=w640, "Message Data"="A", "Message"="cumplimiento", "Message Queue"=w626) -> ("error out"=w627:errorcluster)  [unwired: 6 in, 1 out]
      }
      frame "ingresaMedicionesC" {
        n348 = Flush Queue(queue=w648, error in (no error)=w656) -> (queue out=w645:refnum<queue>, error out=w655:errorcluster)  [unwired: 1 out]
        n349 = Variant To Data(error in=w655, type=string[][] [] ("NewVal"), Variant=w647) -> (data=w658:string[][], error out=w660:errorcluster)
        n350 = Unbundle By Name(w654) -> ("Tabla_C"=w653:string[][], "mediciones"=w650:T7)
        n351 = control-ref of="Tabla_C"() -> (w657:refnum<vi>)
        n352 = call "ingresaMediciones.vi"("New Value"=w658, "Tbl Refnum"=w657, "error in (no error)"=w660, "mediciones in"=w650, "Tabla in"=w653) -> ("error out"=w659:errorcluster, "mediciones out"=w649:T7, "Tabla out"=w651:string[][])  [unwired: 3 in, 1 out]
        n353 = call-poly "Enqueue Message.vi"("error in (no error)"=w659, "Message Data"="C", "Message"="cumplimiento", "Message Queue"=w645) -> ("error out"=w646:errorcluster)  [unwired: 6 in, 1 out]
        n354 = Bundle By Name(cluster=w654, "Tabla_C"=w651, "mediciones"=w649) -> (w652:refnum<class "Prueba04.lvclass">)
      }
      frame "ingresaMedicionesZ" {
        n355 = Flush Queue(queue=w667, error in (no error)=w675) -> (queue out=w664:refnum<queue>, error out=w674:errorcluster)  [unwired: 1 out]
        n356 = Variant To Data(error in=w674, type=string[][] [] ("NewVal"), Variant=w666) -> (data=w677:string[][], error out=w679:errorcluster)
        n357 = Unbundle By Name(w673) -> ("Tabla_Z"=w672:string[][], "mediciones"=w669:T7)
        n358 = control-ref of="Tabla_Z"() -> (w676:refnum<vi>)
        n359 = call "ingresaMediciones.vi"("New Value"=w677, "Tbl Refnum"=w676, "error in (no error)"=w679, "mediciones in"=w669, "Tabla in"=w672) -> ("error out"=w678:errorcluster, "mediciones out"=w668:T7, "Tabla out"=w670:string[][])  [unwired: 3 in, 1 out]
        n360 = Bundle By Name(cluster=w673, "Tabla_Z"=w670, "mediciones"=w668) -> (w671:refnum<class "Prueba04.lvclass">)
        n361 = call-poly "Enqueue Message.vi"("error in (no error)"=w678, "Message Data"="Z", "Message"="cumplimiento", "Message Queue"=w664) -> ("error out"=w665:errorcluster)  [unwired: 6 in, 1 out]
      }
      frame "cumplimiento" {
        n362 = Variant To Data(error in=w695, type="", Variant=w685) -> (data=w688:string, error out=w694:errorcluster)
        n363 = case shown="\"A\", Default" w688 {
          tunnel: w689 -> [w714 w717 w720]
          tunnel: [w713 w716 w719] -> w692
          tunnel: [w712 w715 w718] -> w687
          frame "A", Default {
            n364 = Unbundle By Name(w714) -> ("Tabla_A"=w713:string[][], "mediciones"=w712:T7)
          }
          frame "C" {
            n365 = Unbundle By Name(w717) -> ("Tabla_C"=w716:string[][], "mediciones"=w715:T7)
          }
          frame "Z" {
            n366 = Unbundle By Name(w720) -> ("Tabla_Z"=w719:string[][], "mediciones"=w718:T7)
          }
        }
        n367 = call "cumplimiento.vi"("error in (no error)"=w694, "mediciones in"=w687, "Tabla in"=w692) -> ("error out"=w693:errorcluster, "mediciones out"=w686:T7, "Tabla out"=w691:string[][])  [unwired: 5 in, 1 out]
        n368 = case shown="\"C\"" w688 {
          tunnel: ["C2" "Z2" "A2"] -> w681
          tunnel: w691 -> [w698 w703 w708]
          tunnel: w689 -> [w700 w705 w710]
          tunnel: [w699 w704 w709] -> w690
          tunnel: w686 -> [w697 w702 w707]
          frame "C" {
            n369 = local write "Tabla_C"(w698) -> ()
            n370 = Bundle By Name(cluster=w700, "Tabla_C"=w698, "mediciones"=w697) -> (w699:refnum<class "Prueba04.lvclass">)
          }
          frame "Z" {
            n371 = local write "Tabla_Z"(w703) -> ()
            n372 = Bundle By Name(cluster=w705, "Tabla_Z"=w703, "mediciones"=w702) -> (w704:refnum<class "Prueba04.lvclass">)
          }
          frame "A", Default {
            n373 = local write "Tabla_A"(w708) -> ()
            n374 = Bundle By Name(cluster=w710, "Tabla_A"=w708, "mediciones"=w707) -> (w709:refnum<class "Prueba04.lvclass">)
          }
        }
        n375 = call-poly "Enqueue Message.vi"("error in (no error)"=w693, "Message Data"=w681, "Message"="listo_evaluar", "Message Queue"=w683) -> ("error out"=w684:errorcluster)  [unwired: 6 in, 1 out]
      }
      frame "listo_evaluar" {
        # "si son todos\ndistntos a cero\nentonces todos se\nhan evaluado"
        n376 = Variant To Data(error in=w728, type="" ("y"), Variant=w722) -> (data=w724:string, error out=w726:errorcluster)
        n377 = case shown="\"Z2\"" w724 {
          tunnel: [w734 w760 w786] -> w727
          tunnel: w726 -> [w733 w759 w785]
          tunnel: w723 -> [w732 w758 w784]
          tunnel: w721 -> [w730 w756 w782]
          frame "A2", Default {
            n378 = Unbundle By Name(w732) -> ("Tabla_A"=w731:string[][])
            n379 = Index Array(array=w731, index (col)=8 ("disabled index (col)")) -> (element=w736:string[])  [unwired: 1 in]
            n380 = for {
              tunnel: [w754] -> w735 mode=indexing
              tunnel: w736 -> [w752] mode=indexing
              n381 = Not Equal?(x=w752, y="--") -> (x != y?=w754:bool)
            }
            n382 = And Array Elements(Boolean array=w735) -> (logical AND=w729:bool)
            n383 = case shown="False" w729 {
              tunnel: [w739 w751] -> w734
              tunnel: w733 -> [w741 w750]
              tunnel: w730 -> [w740 w748]
              frame False {
                n384 = local read "generarA2"() -> (w738:bool)
                n385 = case shown="True" w738 {
                  tunnel: w741 -> [w742 w746]
                  tunnel: [w742 w745] -> w739
                  tunnel: w740 -> [_ w744]
                  frame False {
                  }
                  frame True {
                    n386 = call-poly "Enqueue Message.vi"("error in (no error)"=w746, "Message"="Leer_Voltaje", "Message Queue"=w744) -> ("error out"=w745:errorcluster)  [unwired: 7 in, 1 out]
                  }
                }
              }
              frame True {
                n387 = call-poly "Enqueue Message.vi"("error in (no error)"=w750, "Message Data"="A2" ("y"), "Message"="evaluar" ("y"), "Message Queue"=w748) -> ("error out"=w751:errorcluster)  [unwired: 6 in, 1 out]
              }
            }
          }
          frame "C2" {
            n388 = Unbundle By Name(w758) -> ("Tabla_C"=w757:string[][])
            n389 = Index Array(array=w757, index (col)=8 ("disabled index (col)")) -> (element=w762:string[])  [unwired: 1 in]
            n390 = for {
              tunnel: [w780] -> w761 mode=indexing
              tunnel: w762 -> [w778] mode=indexing
              n391 = Not Equal?(x=w778, y="--") -> (x != y?=w780:bool)
            }
            n392 = And Array Elements(Boolean array=w761) -> (logical AND=w755:bool)
            n393 = case shown="True" w755 {
              tunnel: [w765 w777] -> w760
              tunnel: w759 -> [w767 w776]
              tunnel: w756 -> [w766 w774]
              frame False {
                n394 = local read "generarC2"() -> (w764:bool)
                n395 = case shown="False" w764 {
                  tunnel: w767 -> [w768 w772]
                  tunnel: [w768 w771] -> w765
                  tunnel: w766 -> [_ w769]
                  frame False {
                  }
                  frame True {
                    n396 = call-poly "Enqueue Message.vi"("error in (no error)"=w772, "Message"="Leer_Voltaje", "Message Queue"=w769) -> ("error out"=w771:errorcluster)  [unwired: 7 in, 1 out]
                  }
                }
              }
              frame True {
                n397 = call-poly "Enqueue Message.vi"("error in (no error)"=w776, "Message Data"="C2" ("y"), "Message"="evaluar" ("y"), "Message Queue"=w774) -> ("error out"=w777:errorcluster)  [unwired: 6 in, 1 out]
              }
            }
          }
          frame "Z2" {
            n398 = Unbundle By Name(w784) -> ("Tabla_Z"=w783:string[][])
            n399 = Index Array(array=w783, index (col)=8 ("disabled index (col)")) -> (element=w788:string[])  [unwired: 1 in]
            n400 = for {
              tunnel: [w806] -> w787 mode=indexing
              tunnel: w788 -> [w804] mode=indexing
              n401 = Not Equal?(x=w804, y="--") -> (x != y?=w806:bool)
            }
            n402 = And Array Elements(Boolean array=w787) -> (logical AND=w781:bool)
            n403 = case shown="False" w781 {
              tunnel: [w792 w803] -> w786
              tunnel: w785 -> [w793 w802]
              tunnel: w782 -> [w791 w801]
              frame False {
                n404 = local read "generarZ2"() -> (w790:bool)
                n405 = case shown="True" w790 {
                  tunnel: w793 -> [w794 w798]
                  tunnel: [w794 w797] -> w792
                  tunnel: w791 -> [_ w796]
                  frame False {
                  }
                  frame True {
                    n406 = call-poly "Enqueue Message.vi"("error in (no error)"=w798, "Message"="Leer_Voltaje", "Message Queue"=w796) -> ("error out"=w797:errorcluster)  [unwired: 7 in, 1 out]
                  }
                }
              }
              frame True {
                n407 = call-poly "Enqueue Message.vi"("error in (no error)"=w802, "Message Data"="Z2" ("y"), "Message"="evaluar" ("y"), "Message Queue"=w801) -> ("error out"=w803:errorcluster)  [unwired: 6 in, 1 out]
              }
            }
          }
        }
      }
      frame "evaluar" {
        n408 = Variant To Data(error in=w815, type="" ("y"), Variant=w809) -> (data=w811:string, error out=w813:errorcluster)
        n409 = case shown="\"C2\"" w811 {
          tunnel: w810 -> [_ w817 w826 w835]
          frame "False", Default {
          }
          frame "A2" {
            # "si todos cumpln\nentonces el ensayo\ncumple"
            n410 = Unbundle By Name(w817) -> ("Tabla_A"=w816:string[][])
            n411 = Index Array(array=w816, index (col)=8 ("disabled index (col)")) -> (element=w819:string[])  [unwired: 1 in]
            n412 = for {
              tunnel: [w824] -> w820 mode=indexing
              tunnel: w819 -> [w822] mode=indexing
              n413 = Equal?(x=w822, y="Cumple") -> (x = y?=w824:bool)
            }
            n414 = And Array Elements(Boolean array=w820) -> (logical AND=→"cumple_no_cumple_A":bool)
          }
          frame "C2" {
            # "si todos cumpln\nentonces el ensayo\ncumple"
            n415 = Unbundle By Name(w826) -> ("Tabla_C"=w825:string[][])
            n416 = Index Array(array=w825, index (col)=8 ("disabled index (col)")) -> (element=w828:string[])  [unwired: 1 in]
            n417 = for {
              tunnel: [w833] -> w829 mode=indexing
              tunnel: w828 -> [w831] mode=indexing
              n418 = Equal?(x=w831, y="Cumple") -> (x = y?=w833:bool)
            }
            n419 = And Array Elements(Boolean array=w829) -> (logical AND=→"cumple_no_cumple_C":bool)
          }
          frame "Z2" {
            # "si todos cumpln\nentonces el ensayo\ncumple"
            n420 = Unbundle By Name(w835) -> ("Tabla_Z"=w834:string[][])
            n421 = Index Array(array=w834, index (col)=8 ("disabled index (col)")) -> (element=w837:string[])  [unwired: 1 in]
            n422 = for {
              tunnel: [w842] -> w838 mode=indexing
              tunnel: w837 -> [w840] mode=indexing
              n423 = Equal?(x=w840, y="Cumple") -> (x = y?=w842:bool)
            }
            n424 = And Array Elements(Boolean array=w838) -> (logical AND=→"cumple_no_cumple_Z":bool)
          }
        }
        n425 = call-poly "Enqueue Message.vi"("error in (no error)"=w813, "Message"="final", "Message Queue"=w808) -> ("error out"=w814:errorcluster)  [unwired: 7 in, 1 out]
      }
      frame "final" {
        n426 = local read "cumple_no_cumple_A"() -> (w848:bool)
        "cumple_A" <- w848
        n427 = Not(x=w848) -> (.not. x?=→"no_cumple_A":bool)
        n428 = local read "cumple_no_cumple_Z"() -> (w845:bool)
        "cumple_Z" <- w845
        n429 = local read "cumple_no_cumple_C"() -> (w847:bool)
        "cumple_C" <- w847
        n430 = Not(x=w845) -> (.not. x?=→"no_cumple_Z":bool)
        n431 = Not(x=w847) -> (.not. x?=→"no_cumple_C":bool)
      }
      frame "guardaMedicionesA" {
        # "error"
        # "10"
        # "n° filas"
        n432 = Flush Queue(queue=w853, error in (no error)=w864) -> (queue out=w852:refnum<queue>, error out=w851:errorcluster)  [unwired: 1 out]
        n433 = Unbundle By Name(w859) -> ("Tabla_A"=w858:string[][], "mediciones"=w855:T7)
        n434 = call "FGV_fila.vi"("error in (no error)"=w851, "action"=enum16{"increment", "set_start", "get"}."get") -> ("fila out"=w875:i32)  [unwired: 2 in, 1 out]
        n435 = Unbundle By Name(w855) -> ("Medido"=w874:dbl, "Ref"=w873:dbl)
        n436 = property on="cb_frec_A_2" class="CmbBox"() -> ("Strings[]"=w879:string[])  [unwired: 2 in, 2 out]
        n437 = call "FGV_fila.vi"("error in (no error)"=w851, "action"=enum16{"increment", "set_start", "get"}."increment") -> ("fila out"=w867:i32)  [unwired: 2 in, 1 out]
        n438 = Subtract(x=w874, y=w873) -> (x-y=w861:dbl)
        n439 = Equal?(x=w874, y=0.0) -> (x = y?=w871:bool)
        n440 = case shown="True" w871 {
          frame False {
          }
          frame True {
            n441 = One Button Dialog(message="Ingrese valor medido") -> ()  [unwired: 1 in, 1 out]
          }
        }
        n442 = local write "generarA2"(FALSE ("generar_A_2")) -> ()
        n443 = Index Array(array=w858, index (row)=w867, index (col)=1 ("disabled index (col)")) -> (element=w866:string)
        n444 = Index Array(array=w879, index=w867) -> (element=w880:string)
        n445 = Fract/Exp String To Number(string=w866) -> (number=w881:dbl)  [unwired: 3 in, 1 out]
        n446 = call "escribeEnTablaUnValor.vi"("element"=w861, "fila"=w875, "col"=4, "tabla in"=w858) -> ("tabla out"=w856:string[][])  [unwired: 7 in]
        n447 = property on="cb_frec_A_2" class="CmbBox"("Value"=w880) -> ()  [unwired: 2 in, 2 out]
        n448 = local write "voltaje_A"(w881) -> ()
        n449 = Matrix Size(0:w856) -> (1:w869:i32)  [unwired: 1 out]
        n450 = Bundle By Name(cluster=w855, "Medido"=0.0) -> (w854:T7)
        n451 = Decrement(x=w869) -> (x-1=w868:i32)
        n452 = Less?(x=w868, y=w867) -> (x < y?=w862:bool)
        n453 = case shown="False" w862 {
          tunnel: w851 -> [w887 w891]
          tunnel: [w886 w890] -> w863
          tunnel: w852 -> [w885 w889]
          frame False {
            n454 = call-poly "Enqueue Message.vi"("error in (no error)"=w887, "Message"="detenerGEN", "Message Queue"=w885) -> ("error out"=w886:errorcluster, "dup Message Queue"=w883:refnum<queue>)  [unwired: 7 in]
            n455 = call-poly "Enqueue Message.vi"("Message"="ConfigurarGEN_A2", "Message Queue"=w883) -> ()  [unwired: 8 in, 2 out]
          }
          frame True {
            n456 = call-poly "Enqueue Message.vi"("error in (no error)"=w891, "Message"="ultimaFrec", "Message Queue"=w889) -> ("error out"=w890:errorcluster)  [unwired: 7 in, 1 out]
          }
        }
        n457 = Bundle By Name(cluster=w859, "Tabla_A"=w856, "mediciones"=w854) -> (w857:refnum<class "Prueba04.lvclass">)
      }
      frame "guardaMedicionesC" {
        # "error"
        # "10"
        # "n° filas"
        n458 = Unbundle By Name(w899) -> ("Tabla_C"=w898:string[][], "mediciones"=w895:T7)
        n459 = call "FGV_fila.vi"("action"=enum16{"increment", "set_start", "get"}."get") -> ("fila out"=w915:i32)  [unwired: 3 in, 1 out]
        n460 = Unbundle By Name(w895) -> ("Medido"=w914:dbl, "Ref"=w913:dbl)
        n461 = property on="cb_frec_C_2" class="CmbBox"() -> ("Strings[]"=w919:string[])  [unwired: 2 in, 2 out]
        n462 = call "FGV_fila.vi"("action"=enum16{"increment", "set_start", "get"}."increment") -> ("fila out"=w907:i32)  [unwired: 3 in, 1 out]
        n463 = Subtract(x=w914, y=w913) -> (x-y=w901:dbl)
        n464 = Equal?(x=w914, y=0.0) -> (x = y?=w911:bool)
        n465 = case shown="False" w911 {
          frame False {
          }
          frame True {
            n466 = One Button Dialog(message="Ingrese valor medido") -> ()  [unwired: 1 in, 1 out]
          }
        }
        n467 = Index Array(array=w898, index (row)=w907, index (col)=1 ("disabled index (col)")) -> (element=w906:string)
        n468 = Index Array(array=w919, index=w907) -> (element=w920:string)
        n469 = Fract/Exp String To Number(string=w906) -> (number=w921:dbl)  [unwired: 3 in, 1 out]
        n470 = local write "generarC2"(FALSE ("generar_A_2")) -> ()
        n471 = call "escribeEnTablaUnValor.vi"("element"=w901, "fila"=w915, "col"=4, "tabla in"=w898) -> ("tabla out"=w896:string[][])  [unwired: 7 in]
        n472 = property on="cb_frec_C_2" class="CmbBox"("Value"=w920) -> ()  [unwired: 2 in, 2 out]
        n473 = local write "voltaje_C"(w921) -> ()
        n474 = Matrix Size(0:w896) -> (1:w909:i32)  [unwired: 1 out]
        n475 = Bundle By Name(cluster=w895, "Medido"=0.0) -> (w894:T7)
        n476 = Decrement(x=w909) -> (x-1=w908:i32)
        n477 = Less?(x=w908, y=w907) -> (x < y?=w902:bool)
        n478 = case shown="False" w902 {
          tunnel: w904 -> [w927 w931]
          tunnel: [w926 w930] -> w903
          tunnel: w893 -> [w925 w929]
          frame False {
            n479 = call-poly "Enqueue Message.vi"("error in (no error)"=w927, "Message"="detenerGEN", "Message Queue"=w925) -> ("error out"=w926:errorcluster, "dup Message Queue"=w923:refnum<queue>)  [unwired: 7 in]
            n480 = call-poly "Enqueue Message.vi"("Message"="ConfigurarGEN_C2", "Message Queue"=w923) -> ()  [unwired: 8 in, 2 out]
          }
          frame True {
            n481 = call-poly "Enqueue Message.vi"("error in (no error)"=w931, "Message"="ultimaFrec", "Message Queue"=w929) -> ("error out"=w930:errorcluster)  [unwired: 7 in, 1 out]
          }
        }
        n482 = Bundle By Name(cluster=w899, "Tabla_C"=w896, "mediciones"=w894) -> (w897:refnum<class "Prueba04.lvclass">)
      }
      frame "guardaMedicionesZ" {
        # "error"
        # "10"
        # "n° filas"
        n483 = Unbundle By Name(w939) -> ("Tabla_Z"=w938:string[][], "mediciones"=w935:T7)
        n484 = call "FGV_fila.vi"("action"=enum16{"increment", "set_start", "get"}."get") -> ("fila out"=w955:i32)  [unwired: 3 in, 1 out]
        n485 = Unbundle By Name(w935) -> ("Medido"=w954:dbl, "Ref"=w953:dbl)
        n486 = local write "generarZ2"(FALSE ("generar_A_2")) -> ()
        n487 = property on="cb_frec_Z_2" class="CmbBox"() -> ("Strings[]"=w959:string[])  [unwired: 2 in, 2 out]
        n488 = call "FGV_fila.vi"("action"=enum16{"increment", "set_start", "get"}."increment") -> ("fila out"=w947:i32)  [unwired: 3 in, 1 out]
        n489 = Subtract(x=w954, y=w953) -> (x-y=w941:dbl)
        n490 = Equal?(x=w954, y=0.0) -> (x = y?=w951:bool)
        n491 = case shown="True" w951 {
          frame False {
          }
          frame True {
            n492 = One Button Dialog(message="Ingrese valor medido") -> ()  [unwired: 1 in, 1 out]
          }
        }
        n493 = Index Array(array=w938, index (row)=w947, index (col)=1 ("disabled index (col)")) -> (element=w946:string)
        n494 = Index Array(array=w959, index=w947) -> (element=w960:string)
        n495 = Fract/Exp String To Number(string=w946) -> (number=w961:dbl)  [unwired: 3 in, 1 out]
        n496 = call "escribeEnTablaUnValor.vi"("element"=w941, "fila"=w955, "col"=4, "tabla in"=w938) -> ("tabla out"=w936:string[][])  [unwired: 7 in]
        n497 = property on="cb_frec_Z_2" class="CmbBox"("Value"=w960) -> ()  [unwired: 2 in, 2 out]
        n498 = local write "voltaje_Z"(w961) -> ()
        n499 = Matrix Size(0:w936) -> (1:w949:i32)  [unwired: 1 out]
        n500 = Bundle By Name(cluster=w935, "Medido"=0.0) -> (w934:T7)
        n501 = Decrement(x=w949) -> (x-1=w948:i32)
        n502 = Less?(x=w948, y=w947) -> (x < y?=w942:bool)
        n503 = case shown="False" w942 {
          tunnel: w944 -> [w968 w972]
          tunnel: [w964 w971] -> w943
          tunnel: w933 -> [w967 w970]
          frame False {
            n504 = call-poly "Enqueue Message.vi"("error in (no error)"=w968, "Message"="detenerGEN", "Message Queue"=w967) -> ("error out"=w965:errorcluster, "dup Message Queue"=w963:refnum<queue>)  [unwired: 7 in]
            n505 = call-poly "Enqueue Message.vi"("error in (no error)"=w965, "Message"="ConfigurarGEN_Z2", "Message Queue"=w963) -> ("error out"=w964:errorcluster)  [unwired: 7 in, 1 out]
          }
          frame True {
            n506 = call-poly "Enqueue Message.vi"("error in (no error)"=w972, "Message"="ultimaFrec", "Message Queue"=w970) -> ("error out"=w971:errorcluster)  [unwired: 7 in, 1 out]
          }
        }
        n507 = Bundle By Name(cluster=w939, "Tabla_Z"=w936, "mediciones"=w934) -> (w937:refnum<class "Prueba04.lvclass">)
      }
      frame "ultimaFrec" {
        n508 = call "FGV_fila.vi"("error in (no error)"=w978, "fila_inicial"=0, "action"=enum16{"increment", "set_start", "get"}."set_start") -> ("error out"=w977:errorcluster)  [unwired: 1 in, 1 out]
        n509 = call-poly "Enqueue Message.vi"("error in (no error)"=w977, "Message"="detenerGEN", "Message Queue"=w975) -> ("error out"=w981:errorcluster)  [unwired: 7 in, 1 out]
        n510 = One Button Dialog(message="Ultima frecuencia") -> ()  [unwired: 1 in, 1 out]
      }
      frame "Confirmar Salida" {
        n511 = Two Button Dialog(message="¿Quieres cerrar la aplicación?", 1:"No" ("T button name (\"OK\")"), 2:"Si" ("T button name (\"OK\")")) -> (T button?=w986:bool)
        n512 = case shown="True" w986 {
          tunnel: w984 -> [w991 w998]
          tunnel: [w991 w994] -> w983
          tunnel: w985 -> [_ w996]
          frame False {
          }
          frame True {
            n513 = call-poly "Enqueue Message.vi"("error in (no error)"=w998, "Message"="Detener_Instrumento", "Message Queue"=w996) -> ("error out"=w995:errorcluster, "dup Message Queue"=w993:refnum<queue>)  [unwired: 7 in]
            n514 = call-poly "Enqueue Message.vi"("error in (no error)"=w995, "Message"="Exit", "Message Queue"=w993) -> ("error out"=w994:errorcluster)  [unwired: 7 in, 1 out]
          }
        }
      }
      frame "Exit" {
        w1000 = TRUE
        # "#evangelio Manda a cerrar el EHL"
        # "#evangelio Manda a cerrar todos los Loops"
        n515 = Release Queue(queue=w1005, error in (no error)=w1006) -> (error out=w1010:errorcluster)  [unwired: 1 in, 2 out]
        n516 = Unbundle By Name(w1004) -> ("Control references"=w1011:T6)
        n517 = for {
          tunnel: w1003 -> [w1014] mode=indexing
          tunnel: w1001 -> [w1013]
          tunnel: TRUE -> [w1012]
          n518 = call-poly "Enqueue Message.vi"("Priority Message? (F)"=w1012, "Message"=w1013, "Message Queue"=w1014) -> ()  [unwired: 7 in, 2 out]
        }
        n519 = call "Close All Ref.vi"("error in (no error)"=w1010, "Control references"=w1011) -> ("error out"=w1008:errorcluster)  [unwired: 9 in]
        n520 = call "Fire User Event - Stop.vi"("error in (no error)"=w1008, "Event Data"=w1000, "User Event"="Exit EHL", "User Event in"=w1002) -> ("error out"=w999:errorcluster)  [unwired: 7 in]
      }
      frame "Error" {
        w1022 = T8 1 items=["no dialog", "OK message", "continue or stop message", "OK message + warnings", "continue/stop + warnings"] ("type of dialog (OK msg:1)")
        n521 = Variant To Data(error in=w1018, type=errorcluster {"status"=FALSE, "code"=0, "source"=""} ("error out"), Variant=w1015) -> (data=w1020:errorcluster, error out=w1019:errorcluster)
        n522 = call <vilib>:"Simple Error Handler.vi"("type of dialog (OK msg:1)"=w1022, "error in (no error)"=w1020) -> ()  [unwired: 3 in, 5 out]
        n523 = call-poly "Enqueue Message.vi"("error in (no error)"=w1019, "Message"="Exit", "Message Queue"=w1017) -> ("error out"=w1016:errorcluster)  [unwired: 7 in, 1 out]
      }
      frame Default {
        n524 = xnode "Error Ring"("parameter 0"=w1026) -> ("error out"=w1025:errorcluster)
      }
      frame "--------------------------Contoles---------------------------" {
      }
    }
    n525 = call "Error Handler - Message Handling Loop.vi"("error in (no error)"=w31, "Message Queue"=w29) -> ("dup error in"=w30:errorcluster)  [unwired: 8 in, 1 out]
  }
  n526 = while {
    tunnel: [w1041] -> w22
    shift-right: [w1044] -> _
    shift-left: w18 -> [w1045]
    tunnel: w11 -> [w1043]
    tunnel: w10 -> [w1040]
    stop <- w1039 stop-if-true
    n527 = event shown="[16] <User Event From MHL>: User Event" {
      selector: w1045 -> [_ _ _ _ _ _ _ _ _ _ _ _ _ _ _ _ _ _ _ _ _ _ _ _ _ _ _ _ _ _]
      dyn-events: [_ _ _ _ _ _ _ _ _ _ _ _ _ _ _ _ _ _ _ _ _ _ _ _ _ _ _ _ _ _] -> w1044
      timeout: _ -> [_ _ _ _ _ _ _ _ _ _ _ _ _ _ _ _ _ _ _ _ _ _ _ _ _ _ _ _ _ _]
      tunnel: [w1048 w1054 w1060 w1073 w1080 w1093 w1106 w1117 w1128 w1137 w1140 w1147 w1153 w1161 w1169 w1174 _ w1187 w1194 w1197 w1202 w1207 w1213 w1219 w1234 w1239 w1245 w1255 w1264 w1273] -> w1042
      tunnel: w1043 -> [w1050 w1056 w1062 w1075 w1084 w1096 w1107 w1118 w1129 w1138 w1143 w1148 w1156 w1164 w1172 w1178 _ w1188 w1195 w1199 w1204 w1209 w1217 w1224 w1232 w1240 w1246 w1250 w1260 w1269]
      tunnel: w1040 -> [w1047 w1053 w1059 w1065 w1078 w1090 w1102 w1114 w1125 w1136 w1142 w1146 w1152 w1160 w1168 w1177 _ w1189 w1192 _ _ _ w1215 w1223 w1231 w1237 w1243 w1248 w1257 w1266]
      tunnel: [_ _ _ _ _ _ _ _ _ _ _ _ _ _ _ _ w1180 _ _ _ _ _ _ _ _ _ _ _ _ _] -> w1037
      event "go_A": Value Change {
        # "solo cambia el TAB"
        n528 = event-data() -> ()  [unwired: 1 in, 1 out]
        n529 = property on="Tab" class="TabCtl (strict)"(error in=w1050, "Value"=T1."Page 2" ("Tab_Prueba04")) -> (error out=w1049:errorcluster)  [unwired: 1 in, 1 out]
        n530 = call-poly "Enqueue Message.vi"("error in (no error)"=w1049, "Message"="Inicializar_Instrumento_A", "Message Queue"=w1047) -> ("error out"=w1048:errorcluster)  [unwired: 7 in, 1 out]
      }
      event "go_C": Value Change {
        # "solo cambia el TAB"
        n531 = event-data() -> ()  [unwired: 1 in, 1 out]
        n532 = property on="Tab" class="TabCtl (strict)"(error in=w1056, "Value"=T1."Page 4" ("Tab_Prueba04")) -> (error out=w1055:errorcluster)  [unwired: 1 in, 1 out]
        n533 = call-poly "Enqueue Message.vi"("error in (no error)"=w1055, "Message"="Inicializar_Instrumento_C", "Message Queue"=w1053) -> ("error out"=w1054:errorcluster)  [unwired: 7 in, 1 out]
      }
      event "go_Z": Value Change {
        n534 = event-data() -> ()  [unwired: 1 in, 1 out]
        n535 = property on="Tab" class="TabCtl (strict)"(error in=w1062, "Value"=T1."Page 6" ("Tab_Prueba04")) -> (error out=w1061:errorcluster)  [unwired: 1 in, 1 out]
        n536 = call-poly "Enqueue Message.vi"("error in (no error)"=w1061, "Message"="Inicializar_Instrumento_Z", "Message Queue"=w1059) -> ("error out"=w1060:errorcluster)  [unwired: 7 in, 1 out]
      }
      event "generarA1": Value Change {
        n537 = event-data() -> ("NewVal"=w1076:bool)  [unwired: 1 in]
        n538 = Flush Queue(queue=w1065, error in (no error)=w1075) -> (queue out=w1064:refnum<queue>, error out=w1066:errorcluster)  [unwired: 1 out]
        n539 = Select(t="iniciarGEN_A1" ("message"), s=w1076, f="detenerGEN" ("message")) -> (s? t:f=w1070:string)
        n540 = call-poly "Enqueue Message.vi"("Priority Message? (F)"=TRUE, "error in (no error)"=w1066, "Message Data"="A1" ("message"), "Message"=w1070, "Message Queue"=w1064) -> ("error out"=w1074:errorcluster)  [unwired: 5 in, 1 out]
        n541 = property on="guardar_Vref_A" class="Bool"(error in=w1074, "DisabledEnum"=T3."Enabled" ("Disabled")) -> (error out=w1073:errorcluster)  [unwired: 1 in, 1 out]
      }
      event "generarC1": Value Change {
        n542 = event-data() -> ("NewVal"=w1082:bool)  [unwired: 1 in]
        n543 = Flush Queue(queue=w1078, error in (no error)=w1084) -> (queue out=w1077:refnum<queue>, error out=w1079:errorcluster)  [unwired: 1 out]
        n544 = Select(t="iniciarGEN_C1" ("message"), s=w1082, f="detenerGEN" ("message")) -> (s? t:f=w1086:string)
        n545 = call-poly "Enqueue Message.vi"("error in (no error)"=w1079, "Message Data"="C1" ("message"), "Message"=w1086, "Message Queue"=w1077) -> ("error out"=w1083:errorcluster)  [unwired: 6 in, 1 out]
        n546 = property on="guardar_Vref_C" class="Bool"(error in=w1083, "DisabledEnum"=T3."Enabled" ("Disabled")) -> (error out=w1080:errorcluster)  [unwired: 1 in, 1 out]
      }
      event "generarZ1": Value Change {
        n547 = event-data() -> ("NewVal"=w1094:bool)  [unwired: 1 in]
        n548 = Flush Queue(queue=w1090, error in (no error)=w1096) -> (queue out=w1089:refnum<queue>, error out=w1091:errorcluster)  [unwired: 1 out]
        n549 = Select(t="iniciarGEN_Z1" ("message"), s=w1094, f="detenerGEN" ("message")) -> (s? t:f=w1098:string)
        n550 = call-poly "Enqueue Message.vi"("error in (no error)"=w1091, "Message Data"="Z1" ("message"), "Message"=w1098, "Message Queue"=w1089) -> ("error out"=w1095:errorcluster)  [unwired: 6 in, 1 out]
        n551 = property on="guardar_Vref_Z" class="Bool"(error in=w1095, "DisabledEnum"=T3."Enabled" ("Disabled")) -> (error out=w1093:errorcluster)  [unwired: 1 in, 1 out]
      }
      event "generarA2": Value Change {
        n552 = event-data() -> ("NewVal"=w1105:bool)  [unwired: 1 in]
        n553 = Flush Queue(queue=w1102, error in (no error)=w1107) -> (queue out=w1101:refnum<queue>, error out=w1103:errorcluster)  [unwired: 1 out]
        n554 = Select(t="iniciarGEN_A2" ("message"), s=w1105, f="guardaMedicionesA" ("message")) -> (s? t:f=w1109:string)
        n555 = call-poly "Enqueue Message.vi"("Priority Message? (F)"=TRUE, "error in (no error)"=w1103, "Message Data"="A2" ("message"), "Message"=w1109, "Message Queue"=w1101) -> ("error out"=w1106:errorcluster)  [unwired: 5 in, 1 out]
      }
      event "generarC2": Value Change {
        n556 = event-data() -> ("NewVal"=w1116:bool)  [unwired: 1 in]
        n557 = Flush Queue(queue=w1114, error in (no error)=w1118) -> (queue out=w1113:refnum<queue>, error out=w1115:errorcluster)  [unwired: 1 out]
        n558 = Select(t="iniciarGEN_C2" ("message"), s=w1116, f="guardaMedicionesC" ("message")) -> (s? t:f=w1120:string)
        n559 = call-poly "Enqueue Message.vi"("Priority Message? (F)"=TRUE, "error in (no error)"=w1115, "Message Data"="C2" ("message"), "Message"=w1120, "Message Queue"=w1113) -> ("error out"=w1117:errorcluster)  [unwired: 5 in, 1 out]
      }
      event "generarZ2": Value Change {
        n560 = event-data() -> ("NewVal"=w1127:bool)  [unwired: 1 in]
        n561 = Flush Queue(queue=w1125, error in (no error)=w1129) -> (queue out=w1124:refnum<queue>, error out=w1126:errorcluster)  [unwired: 1 out]
        n562 = Select(t="iniciarGEN_Z2" ("message"), s=w1127, f="guardaMedicionesZ" ("message")) -> (s? t:f=w1131:string)
        n563 = call-poly "Enqueue Message.vi"("Priority Message? (F)"=TRUE, "error in (no error)"=w1126, "Message Data"="Z2" ("message"), "Message"=w1131, "Message Queue"=w1124) -> ("error out"=w1128:errorcluster)  [unwired: 5 in, 1 out]
      }
      event "guardar_Vref_A": Value Change {
        n564 = event-data() -> ()  [unwired: 1 in, 1 out]
        n565 = call-poly "Enqueue Message.vi"("Priority Message? (F)"=TRUE, "error in (no error)"=w1138, "Message"="guardarVrefA", "Message Queue"=w1136) -> ("error out"=w1137:errorcluster)  [unwired: 6 in, 1 out]
      }
      event "guardar_Vref_C": Value Change {
        n566 = event-data() -> ()  [unwired: 1 in, 1 out]
        n567 = call-poly "Enqueue Message.vi"("Priority Message? (F)"=TRUE, "error in (no error)"=w1143, "Message"="guardarVrefC", "Message Queue"=w1142) -> ("error out"=w1140:errorcluster)  [unwired: 6 in, 1 out]
      }
      event "guardar_Vref_Z": Value Change {
        n568 = event-data() -> ()  [unwired: 1 in, 1 out]
        n569 = call-poly "Enqueue Message.vi"("Priority Message? (F)"=TRUE, "error in (no error)"=w1148, "Message"="guardarVrefZ", "Message Queue"=w1146) -> ("error out"=w1147:errorcluster)  [unwired: 6 in, 1 out]
      }
      event Value Change {
        n570 = event-data() -> ()  [unwired: 1 in, 1 out]
        n571 = Divide(x="VoltAjuste_A", y=T2 1000.0) -> (x/y=w1149:T2)
        "IndicadorAjuste_A" <- w1149
        n572 = call-poly "Enqueue Message.vi"("Priority Message? (F)"=TRUE, "error in (no error)"=w1156, "Message Data"=w1149, "Message"="EnviarVoltajeGEN", "Message Queue"=w1152) -> ("error out"=w1153:errorcluster)  [unwired: 5 in, 1 out]
      }
      event Value Change {
        n573 = event-data() -> ()  [unwired: 1 in, 1 out]
        n574 = Divide(x="VoltAjuste_C", y=T2 1000.0) -> (x/y=w1158:T2)
        "IndicadorAjuste_C" <- w1158
        n575 = call-poly "Enqueue Message.vi"("Priority Message? (F)"=TRUE, "error in (no error)"=w1164, "Message Data"=w1158, "Message"="EnviarVoltajeGEN", "Message Queue"=w1160) -> ("error out"=w1161:errorcluster)  [unwired: 5 in, 1 out]
      }
      event Value Change {
        n576 = event-data() -> ()  [unwired: 1 in, 1 out]
        n577 = Divide(x="VoltAjuste_Z", y=T2 1000.0) -> (x/y=w1166:T2)
        "IndicadorAjuste_Z" <- w1166
        n578 = call-poly "Enqueue Message.vi"("Priority Message? (F)"=TRUE, "error in (no error)"=w1172, "Message Data"=w1166, "Message"="EnviarVoltajeGEN", "Message Queue"=w1168) -> ("error out"=w1169:errorcluster)  [unwired: 5 in, 1 out]
      }
      event "ir a resultados_A": Value Change {
        n579 = event-data() -> ()  [unwired: 1 in, 1 out]
        n580 = call-poly "Enqueue Message.vi"("Priority Message? (F)"=TRUE, "error in (no error)"=w1178, "Message"="crea_voltajes_prueba_A", "Message Queue"=w1177) -> ("error out"=w1175:errorcluster)  [unwired: 6 in, 1 out]
        n581 = property on="Tab" class="TabCtl (strict)"(error in=w1175, "Value"=T1."Page 3" ("Tab_Prueba04")) -> (error out=w1174:errorcluster)  [unwired: 1 in, 1 out]
      }
      event User Event {
        n582 = event-data() -> ("User Event"=w1182:string, "Event Data"=w1181:variant)  [unwired: 1 in]
        n583 = case shown="\"Exit EHL\"" w1182 {
          tunnel: w1181 -> [_ w1184]
          tunnel: [_ w1183] -> w1180
          frame Default {
          }
          frame "Exit EHL" {
            # "#evangelio Termina\nla ejecucion del EHL"
            n584 = Variant To Data(type=TRUE, Variant=w1184) -> (data=w1183:bool)  [unwired: 1 in, 1 out]
          }
        }
      }
      event Panel Close? {
        w1186 = TRUE
        n585 = event-data() -> ()  [unwired: 1 in, 1 out]
        n586 = call-poly "Enqueue Message.vi"("Priority Message? (F)"=w1186, "error in (no error)"=w1188, "Message"="Confirmar Salida", "Message Queue"=w1189) -> ("error out"=w1187:errorcluster)  [unwired: 6 in, 1 out]
        n587 = event-data("Discard?"=w1186) -> ()  [unwired: 1 in, 1 out]
      }
      event "ir a resultados_C": Value Change {
        n588 = event-data() -> ()  [unwired: 1 in, 1 out]
        n589 = call-poly "Enqueue Message.vi"("error in (no error)"=w1195, "Message"="crea_voltajes_prueba_C", "Message Queue"=w1192) -> ("error out"=w1193:errorcluster)  [unwired: 7 in, 1 out]
        n590 = property on="Tab" class="TabCtl (strict)"(error in=w1193, "Value"=T1."Page 5" ("Tab_Prueba04")) -> (error out=w1194:errorcluster)  [unwired: 1 in, 1 out]
      }
      event "ir a inicio desde A": Value Change {
        w1200 = TRUE ("ponderacion_A")
        n591 = event-data() -> ()  [unwired: 1 in, 1 out]
        n592 = property on="Tab" class="TabCtl (strict)"(error in=w1199, "Value"=T1."Page 1" ("Tab_Prueba04")) -> (error out=w1198:errorcluster)  [unwired: 1 in, 1 out]
        n593 = property on="estado_ensayo_A" class="Str"(error in=w1198, "Visible"=w1200) -> (error out=w1197:errorcluster)  [unwired: 1 in, 1 out]
        "ponderacion_A" <- w1200
      }
      event "ir a inicio desde C": Value Change {
        w1205 = TRUE ("ponderacion_A")
        n594 = event-data() -> ()  [unwired: 1 in, 1 out]
        n595 = property on="Tab" class="TabCtl (strict)"(error in=w1204, "Value"=T1."Page 1" ("Tab_Prueba04")) -> (error out=w1203:errorcluster)  [unwired: 1 in, 1 out]
        n596 = property on="estado_ensayo_C" class="Str"(error in=w1203, "Visible"=w1205) -> (error out=w1202:errorcluster)  [unwired: 1 in, 1 out]
        "ponderacion_C" <- w1205
      }
      event "ir a inicio desde Z": Value Change {
        w1210 = TRUE ("ponderacion_A")
        n597 = event-data() -> ()  [unwired: 1 in, 1 out]
        n598 = property on="Tab" class="TabCtl (strict)"(error in=w1209, "Value"=T1."Page 1" ("Tab_Prueba04")) -> (error out=w1208:errorcluster)  [unwired: 1 in, 1 out]
        n599 = property on="estado_ensayo_Z" class="Str"(error in=w1208, "Visible"=w1210) -> (error out=w1207:errorcluster)  [unwired: 1 in, 1 out]
        "ponderacion_Z" <- w1210
      }
      event "ir a resultados _Z": Value Change {
        n600 = event-data() -> ()  [unwired: 1 in, 1 out]
        n601 = call-poly "Enqueue Message.vi"("error in (no error)"=w1217, "Message"="crea_voltajes_prueba_Z", "Message Queue"=w1215) -> ("error out"=w1216:errorcluster)  [unwired: 7 in, 1 out]
        n602 = property on="Tab" class="TabCtl (strict)"(error in=w1216, "Value"=T1."Page 7" ("Tab_Prueba04")) -> (error out=w1213:errorcluster)  [unwired: 1 in, 1 out]
      }
      event "seguir": Value Change {
        n603 = event-data() -> ()  [unwired: 1 in, 1 out]
        n604 = local read "cumple_prueba04"() -> (w1225:bool)
        n605 = call-poly "Enqueue Message.vi"("error in (no error)"=w1224, "Message"="Detener_Instrumento", "Message Queue"=w1223) -> ("error out"=w1220:errorcluster, "dup Message Queue"=w1218:refnum<queue>)  [unwired: 7 in]
        n606 = Select(t="Cumple", s=w1225, f="No Cumple") -> (s? t:f=→"resultado":string)
        n607 = call-poly "Enqueue Message.vi"("error in (no error)"=w1220, "Message"="Exit", "Message Queue"=w1218) -> ("error out"=w1219:errorcluster)  [unwired: 7 in, 1 out]
      }
      event "Tabla_A": Value Change {
        n608 = event-data() -> ("NewVal"=w1233:string[][])  [unwired: 1 in]
        n609 = call-poly "Enqueue Message.vi"("Priority Message? (F)"=TRUE, "error in (no error)"=w1232, "Message Data"=w1233, "Message"="ingresaMedicionesA", "Message Queue"=w1231) -> ("error out"=w1234:errorcluster)  [unwired: 5 in, 1 out]
      }
      event "Tabla_C": Value Change {
        n610 = event-data() -> ("NewVal"=w1238:string[][])  [unwired: 1 in]
        n611 = call-poly "Enqueue Message.vi"("Priority Message? (F)"=TRUE, "error in (no error)"=w1240, "Message Data"=w1238, "Message"="ingresaMedicionesC", "Message Queue"=w1237) -> ("error out"=w1239:errorcluster)  [unwired: 5 in, 1 out]
      }
      event "Tabla_Z": Value Change {
        n612 = event-data() -> ("NewVal"=w1244:string[][])  [unwired: 1 in]
        n613 = call-poly "Enqueue Message.vi"("Priority Message? (F)"=TRUE, "error in (no error)"=w1246, "Message Data"=w1244, "Message"="ingresaMedicionesZ", "Message Queue"=w1243) -> ("error out"=w1245:errorcluster)  [unwired: 5 in, 1 out]
      }
      event "cb_frec_A_2": Value Change {
        n614 = event-data() -> ("NewVal"=w1253:string)  [unwired: 1 in]
        n615 = property on="cb_frec_A_2" class="CmbBox"() -> ("Strings[]"=w1254:string[])  [unwired: 2 in, 2 out]
        n616 = Search 1D Array(1D array=w1254, element=w1253) -> (index of element=w1251:i32)  [unwired: 1 in]
        n617 = call "FGV_fila.vi"("error in (no error)"=w1250, "fila_inicial"=w1251, "action"=enum16{"increment", "set_start", "get"}."set_start") -> ("error out"=w1249:errorcluster)  [unwired: 1 in, 1 out]
        n618 = call-poly "Enqueue Message.vi"("error in (no error)"=w1249, "Message"="actualizarVrefA", "Message Queue"=w1248) -> ("error out"=w1255:errorcluster)  [unwired: 7 in, 1 out]
      }
      event "cb_frec_C_2": Value Change {
        n619 = event-data() -> ("NewVal"=w1263:string)  [unwired: 1 in]
        n620 = property on="cb_frec_C_2" class="CmbBox"() -> ("Strings[]"=w1258:string[])  [unwired: 2 in, 2 out]
        n621 = Search 1D Array(1D array=w1258, element=w1263) -> (index of element=w1261:i32)  [unwired: 1 in]
        n622 = call "FGV_fila.vi"("error in (no error)"=w1260, "fila_inicial"=w1261, "action"=enum16{"increment", "set_start", "get"}."set_start") -> ("error out"=w1259:errorcluster)  [unwired: 1 in, 1 out]
        n623 = call-poly "Enqueue Message.vi"("error in (no error)"=w1259, "Message"="actualizarVrefC", "Message Queue"=w1257) -> ("error out"=w1264:errorcluster)  [unwired: 7 in, 1 out]
      }
      event "cb_frec_Z_2": Value Change {
        n624 = event-data() -> ("NewVal"=w1272:string)  [unwired: 1 in]
        n625 = property on="cb_frec_Z_2" class="CmbBox"() -> ("Strings[]"=w1267:string[])  [unwired: 2 in, 2 out]
        n626 = Search 1D Array(1D array=w1267, element=w1272) -> (index of element=w1270:i32)  [unwired: 1 in]
        n627 = call "FGV_fila.vi"("error in (no error)"=w1269, "fila_inicial"=w1270, "action"=enum16{"increment", "set_start", "get"}."set_start") -> ("error out"=w1268:errorcluster)  [unwired: 1 in, 1 out]
        n628 = call-poly "Enqueue Message.vi"("error in (no error)"=w1268, "Message"="actualizarVefZ", "Message Queue"=w1266) -> ("error out"=w1273:errorcluster)  [unwired: 7 in, 1 out]
      }
    }
    n629 = call "Error Handler - Event Handling Loop.vi"("error in (no error)"=w1042, "Message Queue"=w1040) -> ("dup error in"=w1041:errorcluster, "Error?"=w1038:bool)  [unwired: 7 in, 1 out]
    n630 = Or(x=w1037, y=w1038) -> (x .or. y?=w1039:bool)
  }
  n631 = call "Inst_CNT90.vi"("error in"=w4, "All Message Queues in"=w3, "Prueba31 in"=w5) -> ()  [unwired: 8 in, 1 out]
  n632 = call "Inst_DS360.vi"("error in"=w4, "All Message Queues in"=w3, "Prueba04 in"=w5) -> ()  [unwired: 8 in, 1 out]
  n633 = call "Inst_K2002.vi"("error in"=w4, "All Message Queues in"=w3, "Prueba31 in"=w5) -> ()  [unwired: 8 in, 1 out]
  n634 = call-dynamic "CleanUp.vi"("Prueba04 in"=w19) -> ("Prueba04 out"=→"Prueba04 out":refnum<class "Prueba04.lvclass">)  [unwired: 9 in, 1 out]
  n635 = Merge Errors(w22, w21) -> (→"error out":errorcluster)
